vi "TAT_Start.vi"(8 "error In":errorcluster) -> (0 "error out":errorcluster)   [LabVIEW 2017]
uses:
  <vilib>/Utility/error.llb/DialogType.ctl
  Controls/Ass. Loop Control.ctl
  <vilib>/addons/database/Connection.llb/Conn ObjectReference.ctl
  7638e5b4-8d4b-4e71-8911-39d6dd532d8c.vi
  b10198c8-4cf2-4d3c-be81-bfa44f374683.vi
  d2a8d04d-9241-49bb-b773-132ee28ef79b.vi
  f36397dc-6f6c-4e3f-bd29-f8e22a7ab89b.vi
  <vilib>/addons/database/Connection.llb/DB Tools Open Connec (Path).vi
  Global/Global 1.vi
  <vilib>/addons/database/NI_Database_API.lvlib
  <vilib>/Utility/config.llb/NI_LVConfig.lvlib
  user32.dll
panel:
  in  "BARCODE STATION 3":string caption="QR CODE :-"
  out "USER:-":string
  in  "Station Tabs":T1(tab)
  out "PRINT LABEL PICKUP":bool caption="LEAK RESULT:-"
  out "RAREJECTION BIN":bool caption="LEAK RESULT:-"
  out "HBC RH PART SENSOR":bool caption="LEAK RESULT:-"
  out "PY1B RHD RH PART SENSOR":bool caption="LEAK RESULT:-"
  out "PY1B LHD RH PART SENSOR":bool caption="LEAK RESULT:-"
  out "HBC LH PART SENSOR":bool caption="LEAK RESULT:-"
  out "PY1B RHD LH PART SENSOR":bool caption="LEAK RESULT:-"
  out "PY1B LHD LH PART SENSOR":bool caption="LEAK RESULT:-"
  out "AMBIET TEMP MIN":u32
  out "BLINKER CURRENT MAX":u32
  out "TEMP SENSOR MAX":u32
  out "BLINKER CURRENT MIN":u32
  out "TEMP SENSOR MIN":u32
  out "String":string="PARAMETERS"
  out "PART NAME :-":string
  out "QR STATION 3":string caption="QR CODE:-"
  out "PLC STATUS:-":bool
  out "PART No.:-":string
  out "TORISHI CODE:-":string
  out "PROJECT :-":string
  out "CYCLE START:-":bool caption="LEAK RESULT:-"
  out "CYCLE TIME:-":u32
  out "SERIAL NO.:- 2":i32
  out "CYCLE RESULT:-":bool caption="LEAK RESULT:-"
  out "QR STATION 1":string caption="SCAN QR CODE:-"
  out "HARNESS CODE":string
  out "CYCLE STATUS STATION 1":string caption="CYCLE STATUS 1:-"
  out "BLINKER CURRENT OK st 1":u32
  out "TEMP SENSOR st 1":u32
  out "Blinker ct st1":bool caption="LEAK RESULT:-"
  out "Temp Sensor st1":bool caption="LEAK RESULT:-"
  out "AMBIENT TEMP st 1":u32
  out "AVM St1":bool caption="LEAK RESULT:-"
  out "iv3 camera st1":bool caption="LEAK RESULT:-"
  out "SHIFT":u16 caption="SHIFT:-"
  out "GLASS ACTR CT 1 mA st2 MAX":dbl
  out "GLASS ACTR CT 2 mA st2 MAX":dbl
  out "SKY st2  MAX":dbl
  out "INTERNAL (DEG) st2 MAX":dbl
  out "EXTERNAL (DEG) st2 MAX":dbl
  out "GROUND st2 MAX":dbl
  out "POWER FOLD CURENT st2 MAX":dbl
  out "GLASS ACTR CT 1 mA st2 MIN":dbl
  out "GLASS PULL TEST st2 MIN":dbl
  out "GLASS ACTR CT 2 mA st2 MIN":dbl
  out "SKY st2 3 MIN":dbl
  out "INTERNAL (DEG) sT2 MIN":dbl
  out "EXTERNAL (DEG) st2 MIN":dbl
  out "GROUND st2 MIN":dbl
  out "POWER FOLD CURENT st2 MIN":dbl
  out "String 2":string="PARAMETERS"
  out "GLASS ACTR CT 1 mA st2 2":dbl
  out "GLASS PULL TEST st2 2":dbl
  out "GLASS ACTR CT 1 mA st2":bool caption="LEAK RESULT:-"
  out "GLASS PULL TEST st2":bool caption="LEAK RESULT:-"
  out "GLASS ACTR CT 2 mA st 2":dbl
  out "GLASS ACTR CT 2 mA st2":bool caption="LEAK RESULT:-"
  out "SKY st2 2":dbl
  out "INTERNAL (DEG) st2":dbl
  out "SKY st2":bool caption="LEAK RESULT:-"
  out "INTERNAL (DG) st2":bool caption="LEAK RESULT:-"
  out "EXTERNAL (DEG) st2 2":dbl
  out "EXTERNAL (DEG) st2":bool caption="LEAK RESULT:-"
  out "GROUND st 2":dbl
  out "GROUND st2":bool caption="LEAK RESULT:-"
  out "POWER FOLD CURENT st 3":dbl
  out "POWER FOLD CURENT st 2":bool caption="LEAK RESULT:-"
  out "QR STATION 2":string caption="QR CODE:-"
  out "SCAN QR STATION 2":string caption="SCAN QR CODE:-"
  out "CYCLE STATUS STATION 2":string caption="CYCLE STATUS 1:-"
  out "PART No.:- St2":string caption="PART No-"
  out "TORISHI :- St2":string caption="TORISHI-"
  out "PLC STATUS:- 2":bool
  out "PART NAME :- St2":string caption="PART NAME-"
  out "CYCLE RESULT:- St2":bool caption="CYCLE RESULT:-"
  out "SERIAL NO.:- St2":i32 caption="SERIAL NO.:-"
  out "CYCLE TIME:-St2":u32 caption="CYCLE TIME:- 2"
  out "CYCLE START:- St 2":bool caption="LEAK RESULT:-"
  out "PY1B LHD LH PART SENSOR 2":bool caption="LEAK RESULT:-"
  out "PY1B & HBC RH PART VERI SENSR":bool caption="LEAK RESULT:-"
  out "GASKET PRESENT SENSOR 2":bool caption="LEAK RESULT:-"
  out "PY1B LHD RH PART SENSOR 2":bool caption="LEAK RESULT:-"
  out "PY1B & HBC LH PART VERI SENSR":bool caption="LEAK RESULT:-"
  out "GASKET PRESENT SENSOR 1":bool caption="LEAK RESULT:-"
  out "RAREJECTION BIN 2":bool caption="LEAK RESULT:-"
  out "PRINT LABEL PICKUP 2":bool caption="LEAK RESULT:-"
  out "Station 1 Bypass":bool
  out "PACKAGE Qty":string
  out "Scanned Qty  2":string
  out "PREVIOUS BARCODE 2":string[](array[string])
  in  "Model Selection:-":string(combo)
  out "CYCLE STATUS STATION 3":string caption="CYCLE STATUS 2:-"
  out "SCANNED QUANTITY":string
  out "PACKAGED QUANTITY":string
  out "PREVIOUS BARCODE":string
  out "BARCODE STATION 3 only display":string caption="QR CODE :-"
  out "PRN to Print":string
  out "PACKAGE STICKER":string
  in  "Stop":bool
  out "RESULT STATION 1":bool caption="FINAL RESULT:-"
  in  "ASS-Alarms":bool
  out "DATE/TIME":string
  # "Nm"
  # "UNIQUE CIRCLE\nAUTOMATION Pvt Ltd"
  # "MIN"
  # "ACTUAL"
  # "MAX"
  # "RESULT"
  # "AMBIENT TEMP"
  # "AVM"
  # "ARABIC_SIGNAL"
  # "BLINKER CURRENT"
  # "TEMP SENSOR"
  # "ACTUAL"
  # "MIN"
  # "MAX"
  # "RESULT"
  # "GLASS ACTR CT 1 mA"
  # "GLASS PULL TEST"
  # "GLASS ACTR CT 2 mA"
  # "GROUND"
  # "SKY"
  # "INTERNAL (DEG)"
  # "EXTERNAL (DEG)"
  # "POWER FOLD CURENT"
  # "MODEL SELECTION:-"
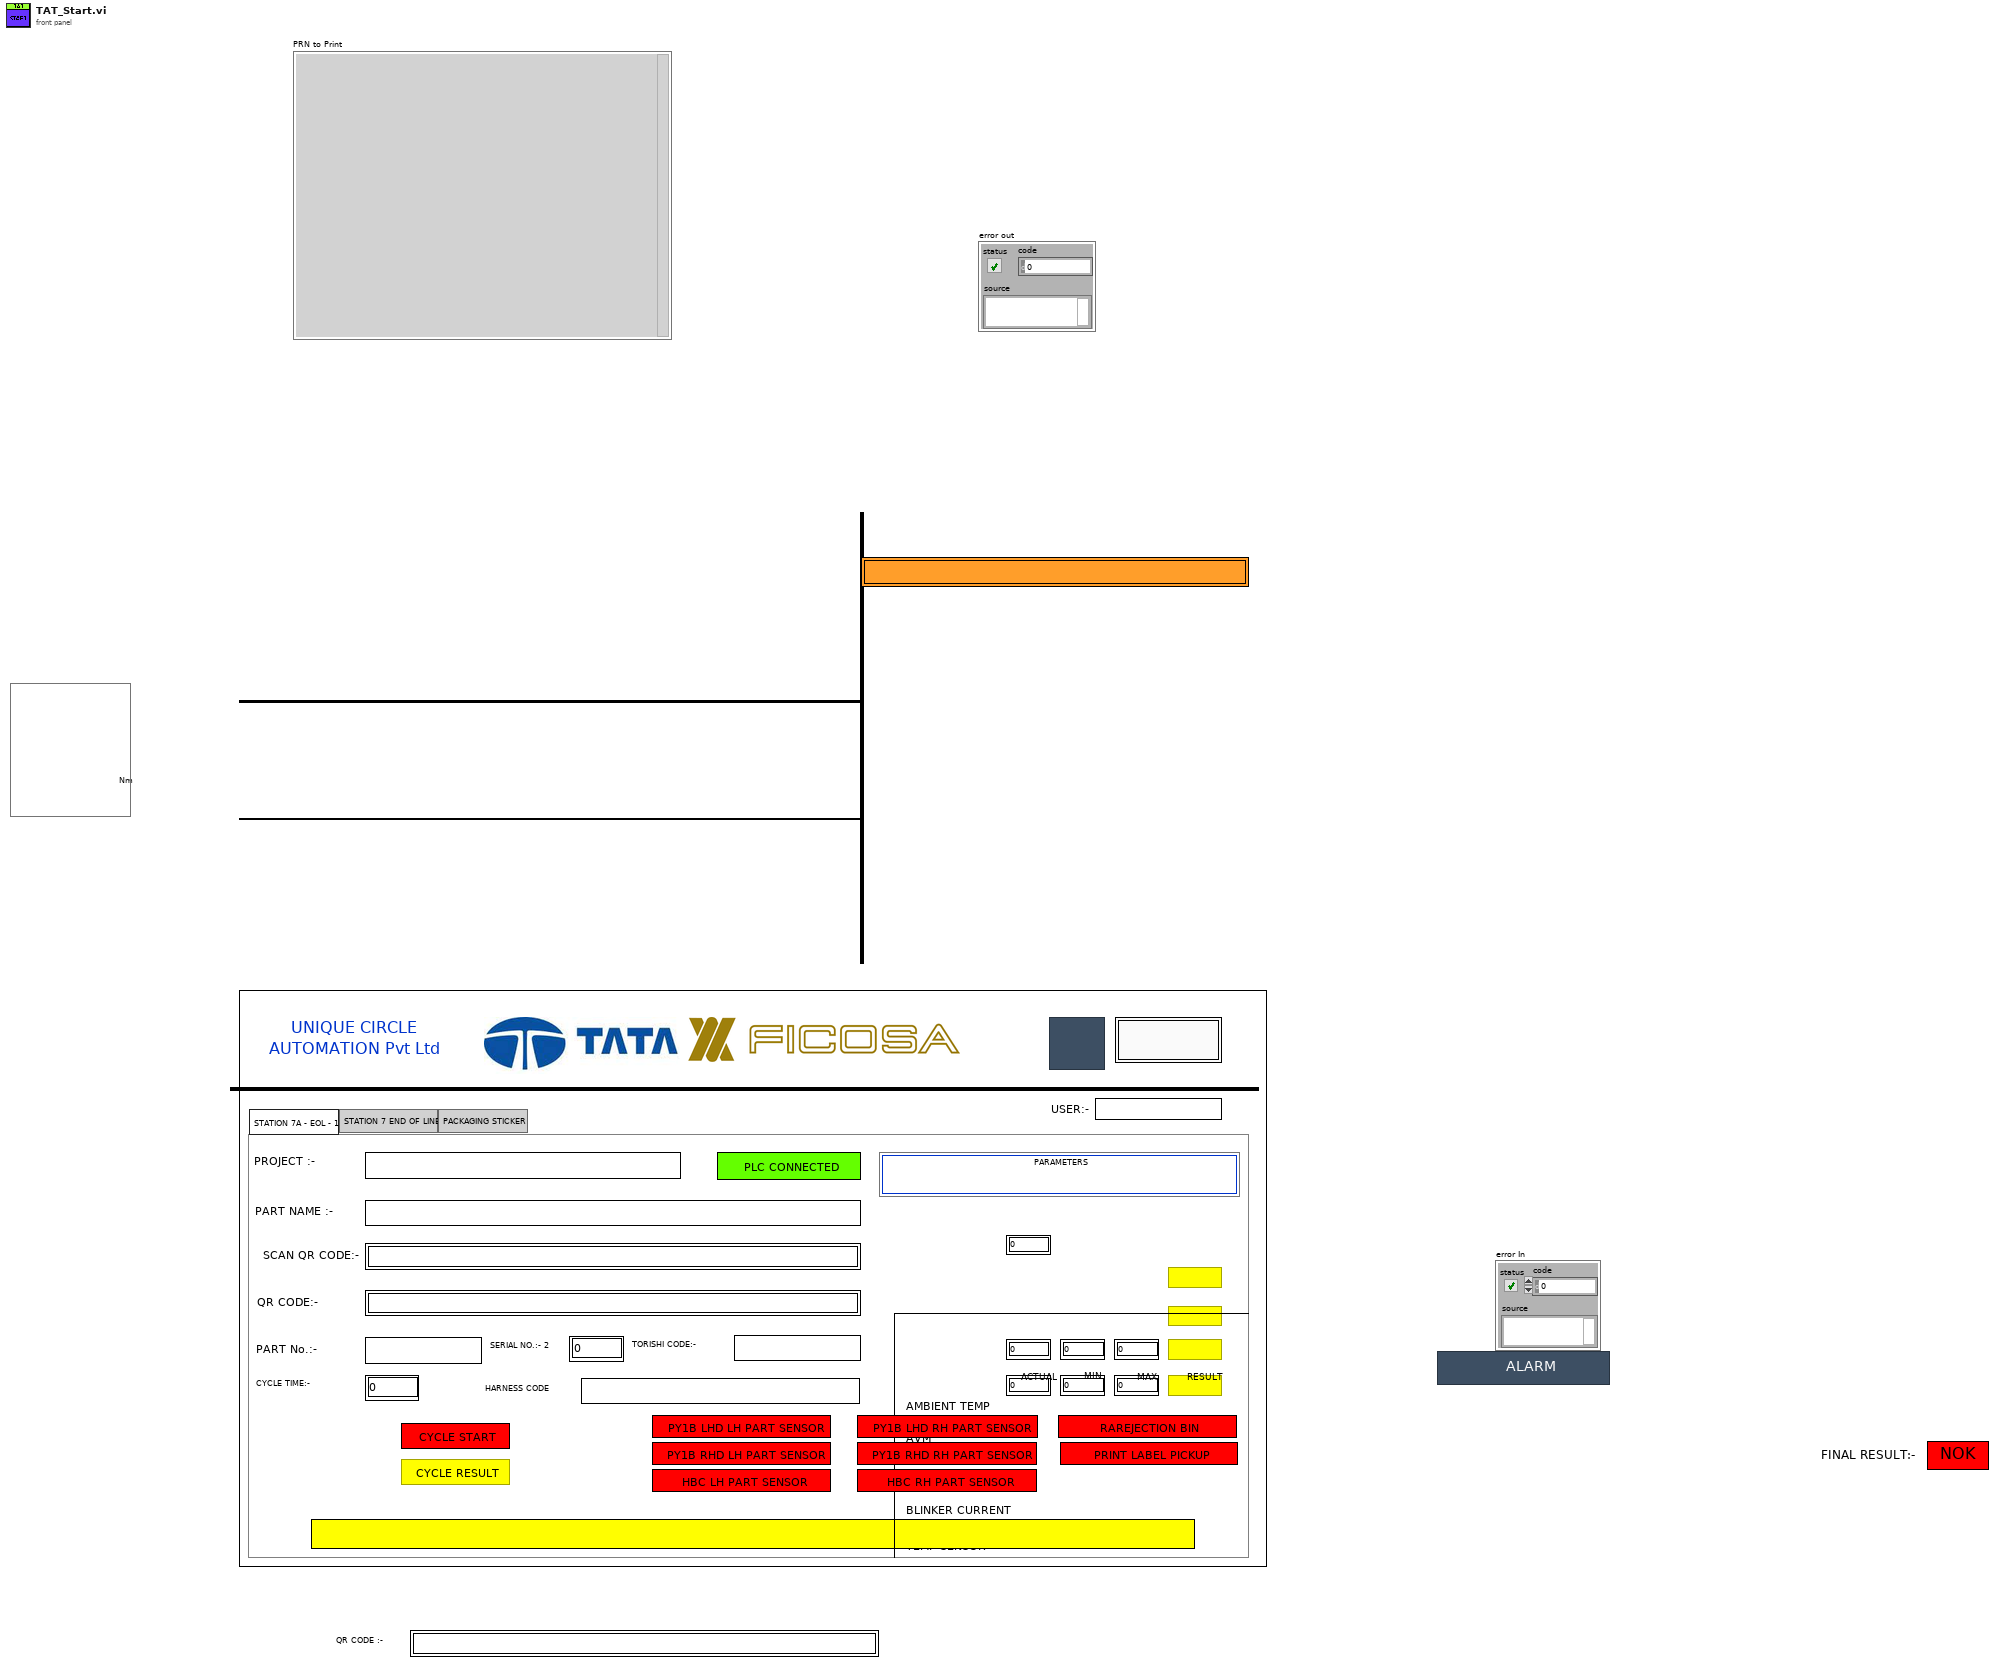
[diagram p1: front panel]
types:
  T1 = enum32{"STATION 7A - EOL - 1", "STATION 7 END OF LINE", "PACKAGING STICKER"}
  T2 = typedef "NI_Database_API.lvlib/Conn ObjectReference.ctl" = refnum<k1>
  T3 = cluster{"Varient number":u16, "Part name":string, "connection reference":T2, "Batch_Size":u16, "PART_NO":string, "TORISHI_CODE":string, "scanner com":refnum<visa-resource-name>, "Part Name List":string[], "Varient path":path, "Current Varient path":path, "Communication path":path, "Package path":path, "Part PRN path":path, "Station2 printer IP":string, "Station1 printer IP":string, "Current Serial Number":string, "Station1_QR":string, "Serial_Number":path, "PREVIOUS code":string[], "Station 2 barcode Dn":string, "Station 2 barcode Up":string, "HARNESS CODE NOT USED":string, "Station 1 bypass":bool}
  T4 = typedef "Ass. Loop Control.ctl" = enum16{"Package_Qty_Count", "GENERATE_QR_PRNT", "Cluster_update", "Waiting_for_scan", "barcode CHECK", "Int", "SaveReport ", "Barcode Print", "Start Cycle", "Wait", "Cycle End", "frontpanel Display update", "Stop"}
  T5 = cluster{"Varient number":u16, "Part name":string, "connection reference":T2, "Batch_Size":u16, "PART_NO":string, "TORISHI_CODE":string, "scanner com":refnum<visa-resource-name>, "Part Name List":string[], "Varient path":path, "Current Varient path":path, "Communication path":path, "Package path":path, "Part PRN path":path, "Station2 printer IP":string, "Station1 printer IP":string, "Current Serial Number":string, "Station2_QR":string, "Serial_Number":path, "PRIVIOUS code":string[], "Barcode station 2 to log Dn":string, "Barcode station 2 to log Up":string, "HARNESS CODE NOT USED":string, "Station1_QR":string, "SearchBitInterlck":bool}
  T6 = cluster{"Varient number":u16, "Part name":string, "Barcode":string, "connection reference":T2, "Batch_Size":u16, "PART_NO":string, "TORISHI_CODE":string, "Varient path":path, "Current Varient path":path, "Communication path":path, "Package path":path, "Part PRN path":path, "Current Serial Number":string, "Station1_QR":string, "Harness_QR_code":string, "SearchBitInterlck":bool}
  T7 = typedef "DialogType.ctl" = u16
  T8 = enum32{"invalid app kind", "Development System", "Run Time System", "Student Edition", "Embedded LabVIEW", "Evaluation", "Custom"}
  T9 = typedef "Semaphore RefNum" = refnum<k1>
  T10 = enum16{"open", "replace", "create", "open or create", "replace or create", "replace or create with confirmation"}
  T11 = cluster{"Varient number":u16, "Part name":string, "connection reference":T2, "Batch_Size":u16, "PART_NO":string, "TORISHI_CODE":string, "scanner com":refnum<visa-resource-name>, "Part Name List":string[], "Varient path":path, "Current Varient path":path, "Communication path":path, "Package path":path, "Part PRN path":path, "Station2 printer IP":string, "Station1 printer IP":string, "Current Serial Number":string, "Station2_QR":string, "Serial_Number":path, "PRIVIOUS code":string[], "Barcode station 2 to log Dn":string, "Barcode station 2 to log Up":string, "HARNESS CODE NOT USED":string, "Station1_QR":string, "searchbitinterlck":bool}
  T12 = typedef "NI_LVConfig.lvlib/Config Data RefNum.ctl" = refnum<k1>
  T13 = cluster{"Varient number":u16, "Part name":string, "Barcode":string, "connection reference":T2, "Batch_Size":u16, "PART_NO":string, "TORISHI_CODE":string, "Varient path":path, "Current Varient path":path, "Communication path":path, "Package path":path, "Part PRN path":path, "Current Serial Number":string, "Station1_QR":string, "Harness_QR_code":string, "searchbitinterlck":bool}
  T14 = cluster{"QR STATION 1":string, "AMBIENT TEMP st 1":u32, "BLINKER CURRENT OK st 1":u32, "TEMP SENSOR st 1":u32}
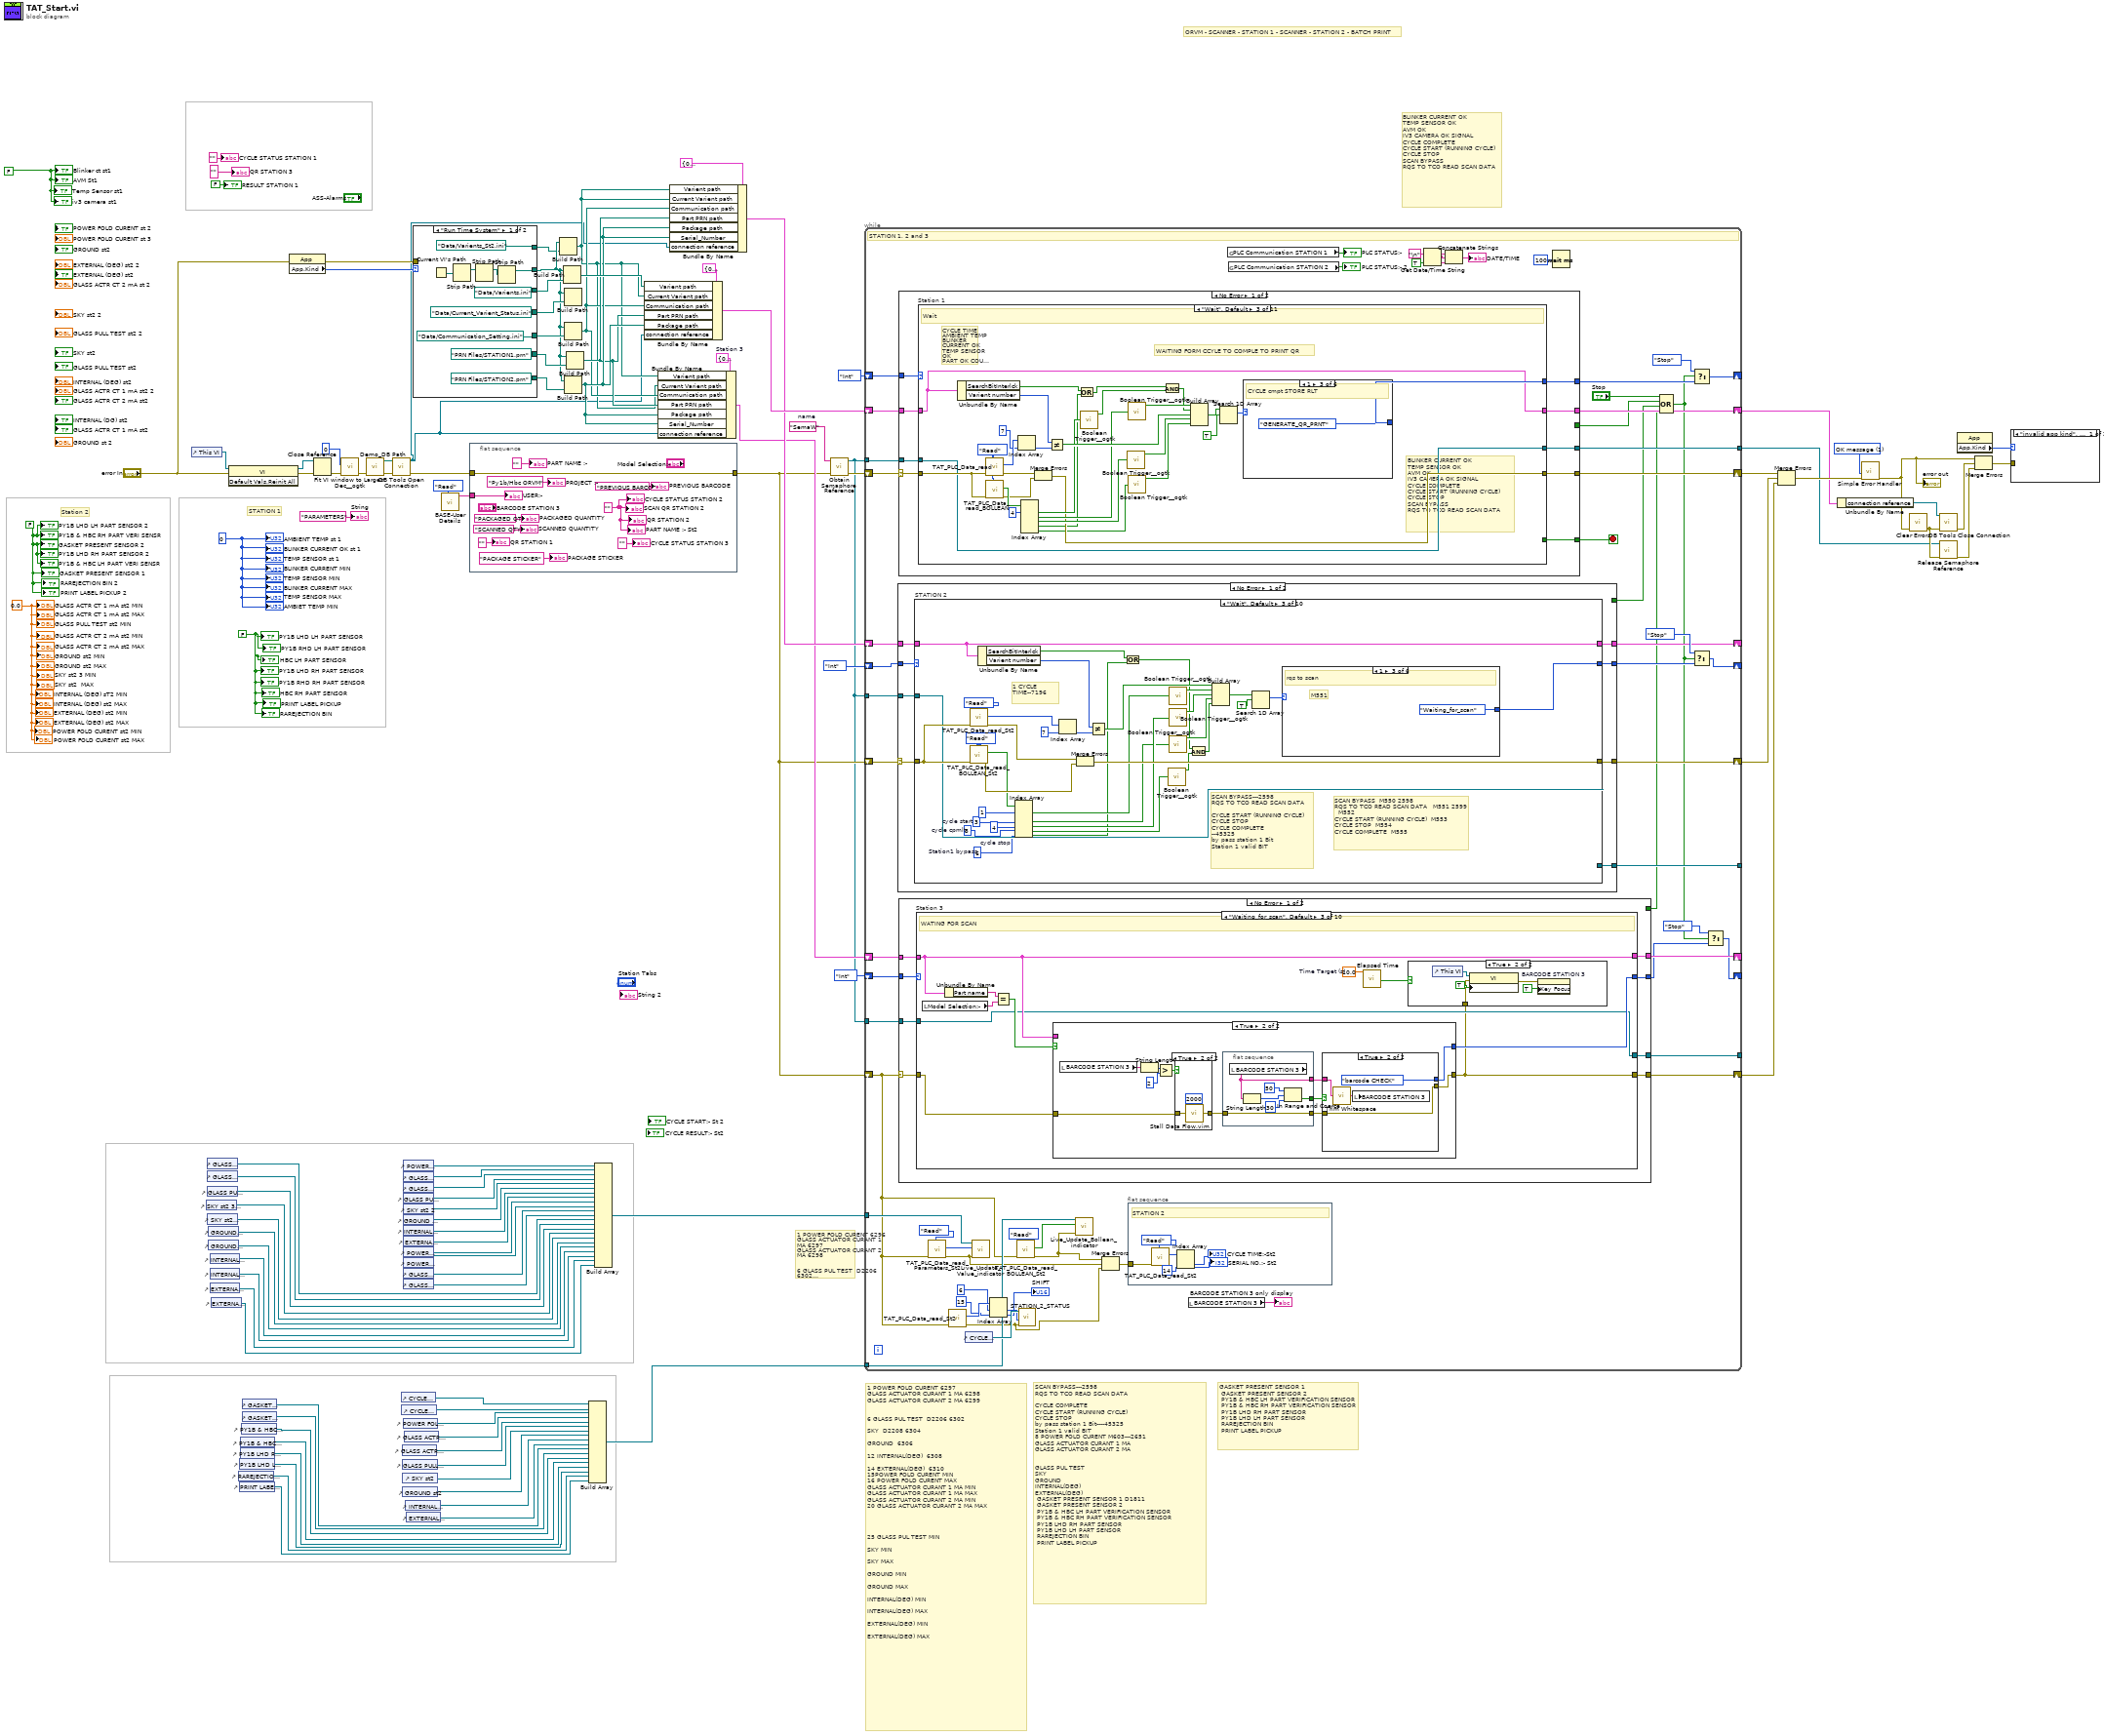
[diagram p0: block diagram]
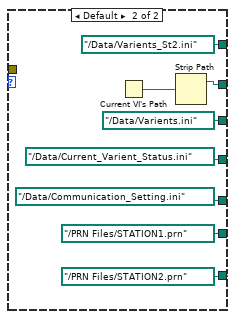
[diagram p2: hidden frame]
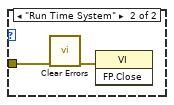
[diagram p3: hidden frame]
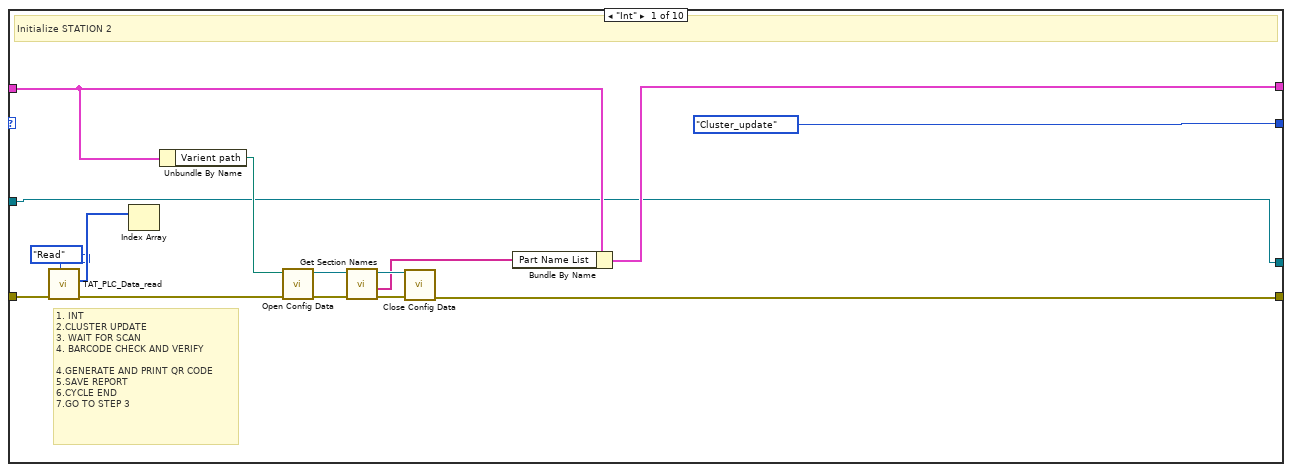
[diagram p4: hidden frame]
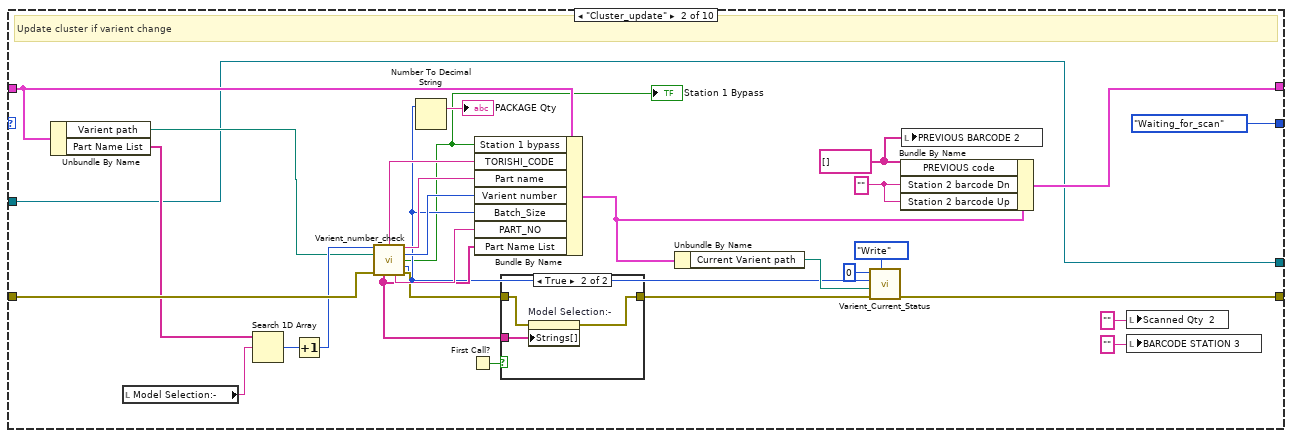
[diagram p5: hidden frame]
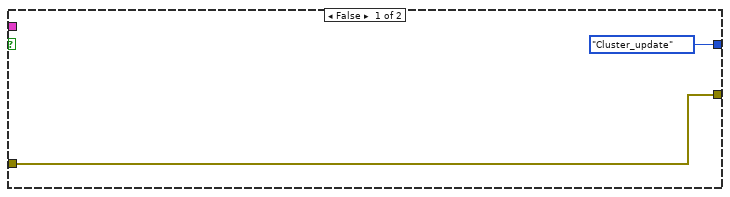
[diagram p8: hidden frame]
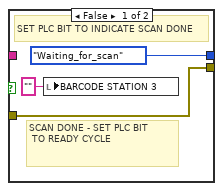
[diagram p10: hidden frame]
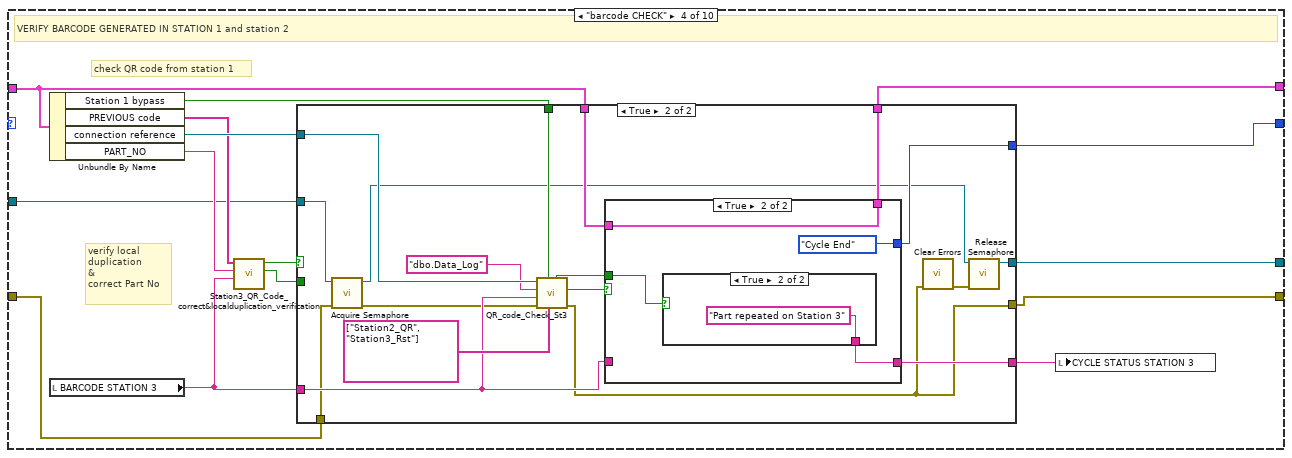
[diagram p11: hidden frame]
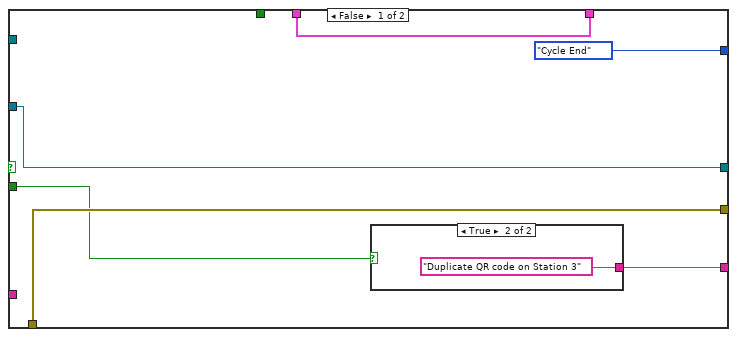
[diagram p12: hidden frame]
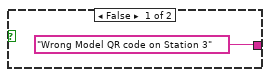
[diagram p13: hidden frame]
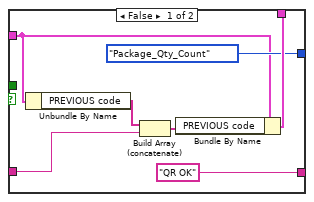
[diagram p14: hidden frame]
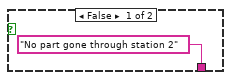
[diagram p15: hidden frame]
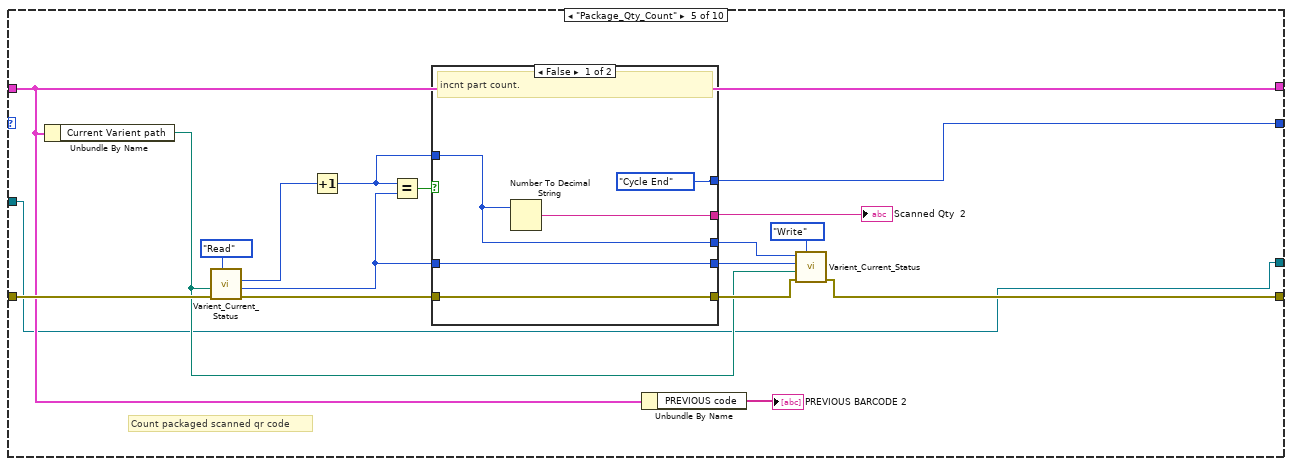
[diagram p16: hidden frame]
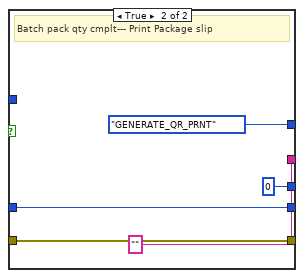
[diagram p17: hidden frame]
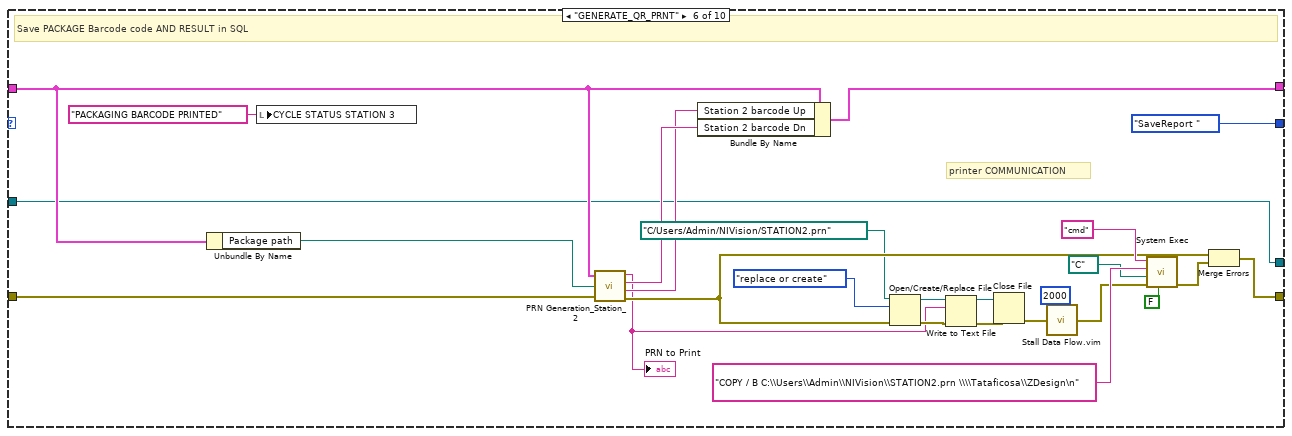
[diagram p18: hidden frame]
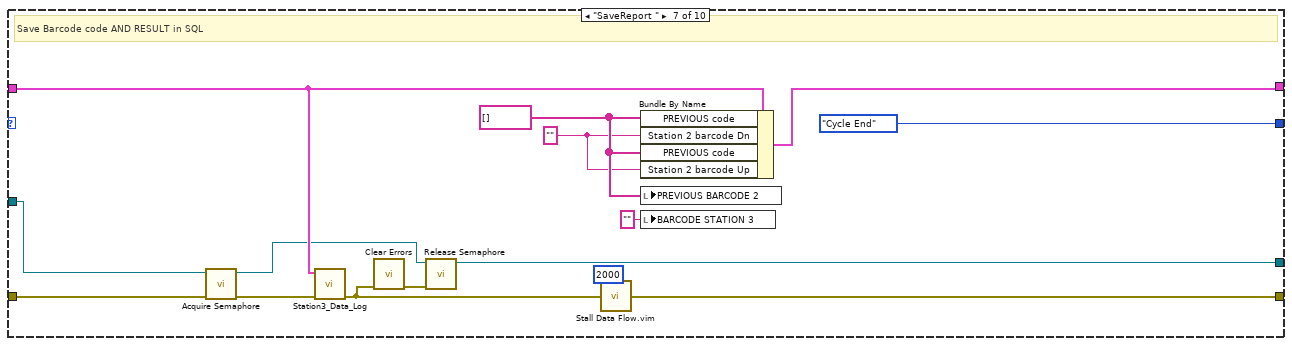
[diagram p19: hidden frame]
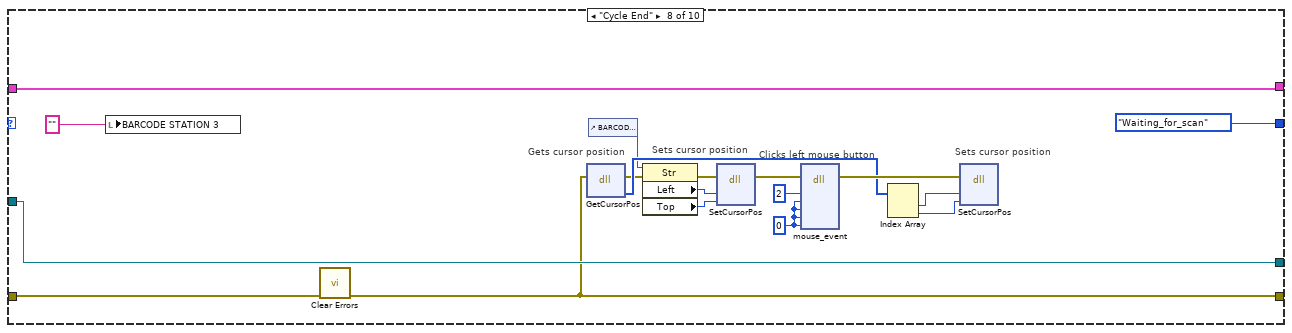
[diagram p20: hidden frame]
diagram:
  w10 = "SemaW"  # name
  w56 = 0.0
  w57 = FALSE
  w58 = FALSE
  w66 = T3 {"Varient number"=0, "Part name"="", "connection reference"=refnum, "Batch_Size"=0, "PART_NO"="", "TORISHI_CODE"="", "scanner com"="", "Part Name List"=[], "Varient path"=path "", "Current Varient path"=path "", "Communication path"=path "", "Package path"=path "", "Part PRN path"=path "", "Station2 printer IP"="", "Station1 printer IP"="", "Current Serial Number"="", "Station1_QR"="", "Serial_Number"=path "", "PREVIOUS code"=[], "Station 2 barcode Dn"="", "Station 2 barcode Up"="", "HARNESS CODE NOT USED"="", "Station 1 bypass"=FALSE}  # Station 3
  w72 = FALSE
  w59 = u32 0 ("AMBIENT TEMP st 1")
  w95 = T7 1 items=["no dialog", "OK message", "continue or stop message", "OK message + warnings", "continue/stop + warnings"] ("type of dialog (OK msg:1)")
  # "GASKET PRESENT SENSOR 1\n GASKET PRESENT SENSOR 2\n PY1B & HBC LH PART VERIFICATION SENSOR\n PY1B & HBC RH PART VERIFICATION SENSOR\n PY1B LHD RH PART SENSOR\n PY1B LHD LH PART SENSOR\n RAREJECTION BIN\n PRINT LABEL PICKUP"
  # "SCAN BYPASS---2598\nRQS TO TCO READ SCAN DATA \n\nCYCLE COMPLETE\nCYCLE START (RUNNING CYCLE)\nCYCLE STOP\nby pass station 1 Bit----45325\nStation 1 valid BIT\n8 POWER FOLD CURENT M603---2651\nGLASS ACTUATOR CURANT 1 MA\nGLASS ACTUATOR CURANT 2 MA\n\n\nGLASS PUL TEST\nSKY \nGROUND\nINTERNAL(DEG)\nEXTERNAL(DEG)\n GASKET PRESENT SENSOR 1 D1811\n GASKET PRESENT SENSOR 2\n PY1B & HBC LH PART VERIFICATION SENSOR\n PY1B & HBC RH PART VERIFICATION SENSOR\n PY1B LHD RH PART SENSOR\n PY1B LHD LH PART SENSOR\n RAREJECTION BIN\n PRINT LABEL PICKUP"
  # "1 POWER FOLD CURENT 6297\nGLASS ACTUATOR CURANT 1 MA 6298\nGLASS ACTUATOR CURANT 2 MA 6299\n\n\n6 GLASS PUL TEST  D2206 6302\n\nSKY  D2208 6304\n\nGROUND  6306\n\n12 INTERNAL(DEG)  6308\n\n14 EXTERNAL(DEG)  6310\n15POWER FOLD CURENT MIN\n16 POWER FOLD CURENT MAX\nGLASS ACTUATOR CURANT 1 MA MIN\nGLASS ACTUATOR CURANT 1 MA MAX\nGLASS ACTUATOR CURANT 2 MA MIN\n20 GLASS ACTUATOR CURANT 2 MA MAX\n\n\n\n\n25 GLASS PUL TEST MIN\n\nSKY MIN\n\nSKY MAX\n\nGROUND MIN\n\nGROUND MAX\n\nINTERNAL(DEG) MIN\n\nINTERNAL(DEG) MAX\n\nEXTERNAL(DEG) MIN\n\nEXTERNAL(DEG) MAX"
  # "Station 2"
  # "STATION 1"
  # "1 POWER FOLD CURENT 6296\nGLASS ACTUATOR CURANT 1 MA 6297\nGLASS ACTUATOR CURANT 2 MA 6298\n\n\n6 GLASS PUL TEST  D2206 6302\n\nSKY  D2208 6304\n\nGROUND  6306\n\n12 INTERNAL(DEG)  6308\n\n14 EXTERNAL(DEG)  6310"
  # "BLINKER CURRENT OK\nTEMP SENSOR OK\nAVM OK\nIV3 CAMERA OK SIGNAL\nCYCLE COMPLETE\nCYCLE START (RUNNING CYCLE)\nCYCLE STOP\nSCAN BYPASS\nRQS TO TCO READ SCAN DATA"
  # "ORVM - SCANNER - STATION 1 - SCANNER - STATION 2 - BATCH PRINT"
  n1 = control-ref of="This VI"() -> (w106:refnum<vi>)
  n2 = control-ref of="SKY st2 3 MIN"() -> (w40:refnum<vi>)
  n3 = control-ref of="GLASS ACTR CT 2 mA st2 MIN"() -> (w43:refnum<vi>)
  n4 = control-ref of="GLASS ACTR CT 2 mA st2 MAX"() -> (w42:refnum<vi>)
  n5 = control-ref of="GLASS PULL TEST st2 MIN"() -> (w41:refnum<vi>)
  n6 = control-ref of="SKY st2  MAX"() -> (w39:refnum<vi>)
  n7 = control-ref of="GROUND st2 MIN"() -> (w38:refnum<vi>)
  n8 = control-ref of="GROUND st2 MAX"() -> (w37:refnum<vi>)
  n9 = control-ref of="INTERNAL (DEG) sT2 MIN"() -> (w36:refnum<vi>)
  n10 = control-ref of="INTERNAL (DEG) st2 MAX"() -> (w35:refnum<vi>)
  n11 = control-ref of="EXTERNAL (DEG) st2 MIN"() -> (w34:refnum<vi>)
  n12 = control-ref of="EXTERNAL (DEG) st2 MAX"() -> (w33:refnum<vi>)
  n13 = invoke class="VI" method="Default Vals.Reinit All"(reference=w106, error in="error In") -> (reference out=w104:refnum<vi>, error out=w105:errorcluster)  [unwired: 1 in, 1 out]
  n14 = control-ref of="RAREJECTION BIN 2"() -> (w15:refnum<vi>)
  n15 = control-ref of="PY1B LHD LH PART SENSOR 2"() -> (w16:refnum<vi>)
  n16 = control-ref of="PRINT LABEL PICKUP 2"() -> (w14:refnum<vi>)
  n17 = control-ref of="PY1B & HBC RH PART VERI SENSR"() -> (w18:refnum<vi>)
  n18 = control-ref of="PY1B LHD RH PART SENSOR 2"() -> (w17:refnum<vi>)
  n19 = control-ref of="PY1B & HBC LH PART VERI SENSR"() -> (w19:refnum<vi>)
  n20 = control-ref of="GASKET PRESENT SENSOR 1"() -> (w21:refnum<vi>)
  n21 = control-ref of="GASKET PRESENT SENSOR 2"() -> (w20:refnum<vi>)
  n22 = property class="App"(error in="error In") -> (error out=w87:errorcluster, "App.Kind"=w92:T8)  [unwired: 1 in, 1 out]
  n23 = Close Reference(reference=w104, error in (no error)=w105) -> (error out=w103:errorcluster)
  n24 = call <userlib>:"Fit VI window to Largest Dec__ogtk.vi"("error in (no error)"=w103, "border spacing (2 px)"=0) -> ("error out"=w80:errorcluster)  [unwired: 4 in, 1 out]
  n25 = call "Demo_DB Path.vi"("error in"=w80) -> ("error out"=w82:errorcluster, "DB Path"=w81:path)  [unwired: 9 in]
  n26 = call-poly <vilib>:"DB Tools Open Connection.vi"("error in (no error)"=w82, "connection information"=w81) -> ("error out"=w4:errorcluster, "connection reference"=w3:T2)  [unwired: 6 in]
  n27 = control-ref of="CYCLE START:- St 2"() -> (w31:refnum<vi>)
  n28 = control-ref of="CYCLE RESULT:- St2"() -> (w30:refnum<vi>)
  n29 = control-ref of="GLASS ACTR CT 2 mA st2"() -> (w27:refnum<vi>)
  n30 = control-ref of="GLASS PULL TEST st2"() -> (w26:refnum<vi>)
  n31 = control-ref of="SKY st2"() -> (w25:refnum<vi>)
  n32 = control-ref of="GROUND st2"() -> (w24:refnum<vi>)
  n33 = control-ref of="POWER FOLD CURENT st 3"() -> (w55:refnum<vi>)
  n34 = control-ref of="GLASS ACTR CT 1 mA st2 2"() -> (w54:refnum<vi>)
  n35 = control-ref of="GLASS ACTR CT 2 mA st 2"() -> (w53:refnum<vi>)
  n36 = control-ref of="GLASS PULL TEST st2 2"() -> (w52:refnum<vi>)
  n37 = control-ref of="SKY st2 2"() -> (w51:refnum<vi>)
  n38 = control-ref of="GROUND st 2"() -> (w50:refnum<vi>)
  n39 = control-ref of="INTERNAL (DEG) st2"() -> (w49:refnum<vi>)
  n40 = control-ref of="EXTERNAL (DEG) st2 2"() -> (w48:refnum<vi>)
  n41 = control-ref of="POWER FOLD CURENT st2 MIN"() -> (w47:refnum<vi>)
  n42 = control-ref of="POWER FOLD CURENT st2 MAX"() -> (w46:refnum<vi>)
  n43 = control-ref of="GLASS ACTR CT 1 mA st2 MIN"() -> (w45:refnum<vi>)
  n44 = control-ref of="GLASS ACTR CT 1 mA st2 MAX"() -> (w44:refnum<vi>)
  n45 = control-ref of="POWER FOLD CURENT st 2"() -> (w29:refnum<vi>)
  n46 = control-ref of="GLASS ACTR CT 1 mA st2"() -> (w28:refnum<vi>)
  n47 = control-ref of="INTERNAL (DG) st2"() -> (w23:refnum<vi>)
  n48 = control-ref of="EXTERNAL (DEG) st2"() -> (w22:refnum<vi>)
  n49 = case shown="\"Run Time System\"" w92 {
    tunnel: [path "Data/Varients.ini" ("path") path "../Data/Varients.ini" ("path")] -> w91
    tunnel: [w112 w122] -> w69
    tunnel: [path "Data/Current_Varient_Status.ini" ("path") path "../Data/Current_Varient_Status.ini" ("path")] -> w90
    tunnel: [path "Data/Communication_Setting.ini" ("path") path "../Data/Communication_Setting.ini" ("path")] -> w89
    tunnel: [path "PRN Files/STATION2.prn" ("path") path "../PRN Files/STATION2.prn" ("path")] -> w88
    tunnel: w87 -> [_ _]
    tunnel: [path "PRN Files/STATION1.prn" ("path") path "../PRN Files/STATION1.prn" ("path")] -> w85
    tunnel: [path "Data/Varients_St2.ini" ("path") path "../Data/Varients_St2.ini" ("path")] -> w68
    frame "Run Time System" {
      n50 = Current VI's Path() -> (path=w115:path)
      n51 = Strip Path(path=w115) -> (stripped path=w114:path)  [unwired: 1 out]
      n52 = Strip Path(path=w114) -> (stripped path=w113:path)  [unwired: 1 out]
      n53 = Strip Path(path=w113) -> (stripped path=w112:path)  [unwired: 1 out]
    }
    frame Default {
      n54 = Current VI's Path() -> (path=w123:path)
      n55 = Strip Path(path=w123) -> (stripped path=w122:path)  [unwired: 1 out]
    }
  }
  n56 = call "BASE-User Details.vi"("Enum"=enum16{"Read", "Write"}."Read") -> ("User Name Out"=w96:string)  [unwired: 9 in, 1 out]
  n57 = flat-sequence {
    tunnel: [w135] -> w12
    tunnel: w4 -> [w135]
    tunnel: w96 -> [w133]
    frame #0 {
      w125 = "" ("BARCODE STATION 2")
      "USER:-" <- w133
      "PART NAME :-" <- ""
      "PROJECT :-" <- "Py1b/Hbc ORVM" ("PROJECT")
      "CYCLE STATUS STATION 3" <- "" ("CYCLE STATUS STATION 2")
      "PACKAGE STICKER" <- "PACKAGE STICKER" ("PACKAGE STICKER")
      "SCANNED QUANTITY" <- "SCANNED QTY" ("PACKAGE STICKER")
      "PACKAGED QUANTITY" <- "PACKAGED QTY" ("PACKAGE STICKER")
      "PREVIOUS BARCODE" <- "PREVIOUS BARCODE" ("PACKAGE STICKER")
      "QR STATION 1" <- "" ("BARCODE STATION 2")
      "SCAN QR STATION 2" <- w125
      "QR STATION 2" <- w125
      "CYCLE STATUS STATION 2" <- w125
      "PART NAME :- St2" <- w125
    }
  }
  n58 = Build Path(base path=w69, name or relative path=w68) -> (appended path=w61:path)
  n59 = Build Path(base path=w69, name or relative path=w91) -> (appended path=w67:path)
  n60 = Build Path(base path=w69, name or relative path=w90) -> ()  [unwired: 1 out]
  n61 = Build Path(base path=w69, name or relative path=w88) -> (appended path=w65:path)
  n62 = Build Path(base path=w69, name or relative path=w89) -> (appended path=w63:path)
  n63 = Build Path(base path=w69, name or relative path=w85) -> (appended path=w64:path)
  n64 = Build Array(w31, w30, w29, w28, w27, w26, w25, w24, w23, w22, w21, w20, w19, w18, w17, w16, w15, w14) -> (w13:refnum<vi>[])
  n65 = Build Array(w55, w54, w53, w52, w51, w50, w49, w48, w47, w46, w45, w44, w43, w42, w41, w40, w39, w38, w37, w36, w35, w34, w33) -> (w32:refnum<vi>[])
  n66 = Bundle By Name(cluster=T6 {"Varient number"=0, "Part name"="", "Barcode"="", "connection reference"=refnum, "Batch_Size"=0, "PART_NO"="", "TORISHI_CODE"="", "Varient path"=path "", "Current Varient path"=path "", "Communication path"=path "", "Package path"=path "", "Part PRN path"=path "", "Current Serial Number"="", "Station1_QR"="", "Harness_QR_code"="", "SearchBitInterlck"=FALSE}, "Varient path"=w67, "Current Varient path"=w61, "Communication path"=w63, "Part PRN path"=w64, "Package path"=w65, "connection reference"=w3) -> (w83:T6)
  n67 = Bundle By Name(cluster=w66, "Varient path"=w61, "Current Varient path"=w61, "Communication path"=w63, "Part PRN path"=w64, "Package path"=w65, "Serial_Number"=w65, "connection reference"=w3) -> (w62:T3)
  n68 = Bundle By Name(cluster=T5 {"Varient number"=0, "Part name"="", "connection reference"=refnum, "Batch_Size"=0, "PART_NO"="", "TORISHI_CODE"="", "scanner com"="", "Part Name List"=[], "Varient path"=path "", "Current Varient path"=path "", "Communication path"=path "", "Package path"=path "", "Part PRN path"=path "", "Station2 printer IP"="", "Station1 printer IP"="", "Current Serial Number"="", "Station2_QR"="", "Serial_Number"=path "", "PRIVIOUS code"=[], "Barcode station 2 to log Dn"="", "Barcode station 2 to log Up"="", "HARNESS CODE NOT USED"="", "Station1_QR"="", "SearchBitInterlck"=FALSE}, "Varient path"=w61, "Current Varient path"=w61, "Communication path"=w63, "Part PRN path"=w64, "Package path"=w65, "Serial_Number"=w65, "connection reference"=w3) -> (w71:T5)
  n69 = call <vilib>:"Obtain Semaphore Reference.vi"("error in (no error)"=w12, "name (unnamed)"=w10) -> ("error out"=w11:errorcluster, "semaphore"=w9:T9)  [unwired: 3 in, 1 out]
  n70 = while {
    shift-right: [w193] -> _
    shift-left: Ass._Loop_Control."Int" ("Enum") -> [w196]
    shift-right: [w180] -> w78
    shift-left: w83 -> [w194]
    shift-right: [w182] -> _
    shift-left: Ass._Loop_Control."Int" ("Enum") -> [w185]
    shift-right: [w183] -> _
    shift-left: w62 -> [w184]
    shift-right: [w175] -> _
    shift-left: Ass._Loop_Control."Int" ("Enum") -> [w178]
    shift-right: [w174] -> _
    shift-left: w71 -> [w173]
    shift-right: [w163] -> w6
    shift-left: w12 -> [w157]
    tunnel: w32 -> [w159]
    tunnel: w13 -> [w158]
    tunnel: w9 -> [w150]
    tunnel: [w149] -> w7
    tunnel: w9 -> [w148]
    tunnel: [w147] -> _
    tunnel: w9 -> [w146]
    tunnel: [w145] -> _
    shift-right: [w151] -> w2
    shift-left: w12 -> [w179]
    shift-right: [w152] -> w1
    shift-left: w11 -> [w139]
    stop <- w186 stop-if-true
    # "STATION 1, 2 and 3"
    n71 = case shown="No Error" w179 {
      selector: w179 -> [w465 w810]
      tunnel: w178 -> [w464 _]
      tunnel: [w463 w813] -> w176
      tunnel: [w462 w814] -> w174
      tunnel: w173 -> [w461 w814]
      tunnel: [w460 w808] -> w151
      tunnel: w148 -> [w459 w812]
      tunnel: [w458 w812] -> w147
      tunnel: [_ TRUE] -> w141
      frame No Error {
        n72 = case "STATION 2" shown="\"Wait\", Default" w464 {
          tunnel: [Ass._Loop_Control."Cluster_update" ("Enum") Ass._Loop_Control."Wait" ("Enum") w529 Ass._Loop_Control."barcode CHECK" ("Enum") w588 Ass._Loop_Control."Wait" ("Enum") Ass._Loop_Control."SaveReport " ("Enum") Ass._Loop_Control."Cycle End" ("Enum") Ass._Loop_Control."Wait" ("Enum") Ass._Loop_Control."Stop" ("Enum")] -> w463
          tunnel: [w487 w502 w530 w573 w575 w706 w717 w745 w754 w802] -> w462
          tunnel: [w483 w506 w542 w557 w585 w689 w716 w738 w761 w785] -> w460
          tunnel: w465 -> [w484 w501 w526 w558 w591 w704 w715 w744 w765 w799]
          tunnel: w461 -> [w487 w505 w530 w573 w584 w706 w725 w745 w755 w802]
          tunnel: w459 -> [w482 w492 w518 w554 w578 w702 w712 w735 w762 w783]
          tunnel: [w482 w492 w518 w554 w577 w702 w712 w733 w762 w783] -> w458
          frame "Int" {
            w466 = enum16{"update", "init"}."init"  # Enum
            w467 = "initia"  # Log data
            # "Keep this on as in first cycle this bit need to be ON.\nRQST FROM TCO RESET SCAN DATA\tM545\t\t\t2593"
            # "SCAN OK\tM542\t\t\t2590\nSCAN NG \tM543\t\t\t2591\nSoftware on Bit\tM544\t\t\t2592\nRQST FROM TCO RESET SCAN DATA\tM545\t\t\t2593\nRepeat scan part\t\tM547\t\t2595\nPass not done station 1\t\tM548\t\t2596"
            # "Initialize STATION 2"
            n73 = control-ref of="CYCLE STATUS STATION 2"() -> (w485:refnum<vi>)
            n74 = call "STATION_2_STATUS.vi"("error in (no error)"=w484, "STATUS"="STATION 7 END OF LINE" ("TexT"), "Ctl Refnum"=w485) -> ("error out"=w469:errorcluster)  [unwired: 8 in]
            n75 = call "TAT_LABVIEW_TO_PLC_St2.vi"("Enum"=enum16{"Read", "Write"}."Read", "error in (no error)"=w469) -> ("error out"=w480:errorcluster, "Array 2"=w473:bool[])  [unwired: 8 in]
            n76 = in-place {
              in-place-border: [w491] -> w481
              in-place-border: w480 -> [w491]
              w490 = FALSE ("element")
              w489 = TRUE ("new element/subarray")
              n77 = in-place-array #1(w473, 0, 1, 2, 3, 4, 5) -> ()  [unwired: 6 out]
              n78 = in-place-array #1(w490, w490, w489, w489, w490, w490) -> (w478:bool[])  [unwired: 6 out]
            }
            n79 = call "TAT_LABVIEW_TO_PLC_St2.vi"("Enum"=enum16{"Read", "Write"}."Write", "error in (no error)"=w481, "Array"=w478) -> ("error out"=w468:errorcluster)  [unwired: 7 in, 1 out]
            n80 = Merge Errors(w468) -> (w483:errorcluster)
            n81 = call "debuglog.vi"("Enum"=w466, "Log data"=w467) -> ()  [unwired: 10 in]
          }
          frame "Cluster_update" {
            # "Update cluster if varient change"
            n82 = call "TAT_PLC_Data_read_St2.vi"("Enum"=enum16{"Read", "Write"}."Read", "error in (no error)"=w501) -> ("error out"=w500:errorcluster, "Array 2"=w497:u16[])  [unwired: 8 in]
            n83 = Unbundle By Name(w505) -> ("Varient path"=w507:path)
            n84 = Index Array(array=w497, index=7) -> (element=w496:u16)
            n85 = call "Varient_number_check.vi"("Varient No."=w496, "Varient path"=w507, "error in"=w500) -> ("TORISHI_CODE"=w494:string, "Part Name"=w493:string, "Varient Number"=w504:i32, "Batch Size"=w503:i32, "PART_NO"=w495:string, "error out"=w506:errorcluster)  [unwired: 4 in, 3 out]
            "PART No.:- St2" <- w495
            "TORISHI :- St2" <- w494
            n86 = local write "PART NAME :- St2"(w493) -> ()
            n87 = Bundle By Name(cluster=w505, "TORISHI_CODE"=w494, "Part name"=w493, "Varient number"=w504, "Batch_Size"=w503, "PART_NO"=w495) -> (w502:T5)
          }
          frame "Wait", Default {
            w511 = 6  # Station1 bypass
            w515 = 5  # cycle cpmlt
            w516 = 4  # cycle stop
            w517 = 3  # cycle start
            # "SCAN BYPASS\t\tM550\t2598\nRQS TO TCO READ SCAN DATA \t\tM551\t2599\n\t\tM552\t\nCYCLE START (RUNNING CYCLE)\t\tM553\t\nCYCLE STOP\t\tM554\t\nCYCLE COMPLETE\t\tM555"
            # "SCAN BYPASS---2598\nRQS TO TCO READ SCAN DATA \n\nCYCLE START (RUNNING CYCLE)\nCYCLE STOP\nCYCLE COMPLETE\n--45325\nby pass station 1 Bit\nStation 1 valid BIT"
            # "1 CYCLE TIME--7196\n\n\n\n\n\n7 FAULT BIT ----4356\nVARIENT\nHOUR\nMINUTE\nSECOND\nDAY\nMONTH\nYEAR\nSERIAL NUMBER\nShift\nPOWER FOLD ACTUATO--D6061\nGLASS ACTUATOR 1 &2"
            n88 = call "TAT_PLC_Data_read_BOLLEAN_St2.vi"("Enum"=enum16{"Read", "Write"}."Read", "error in (no error)"=w526) -> ("error out"=w543:errorcluster, "Array 2"=w522:bool[])  [unwired: 8 in]
            n89 = call "TAT_PLC_Data_read_St2.vi"("Enum"=enum16{"Read", "Write"}."Read", "error in (no error)"=w526) -> ("error out"=w525:errorcluster, "Array 2"=w527:u16[])  [unwired: 8 in]
            n90 = Unbundle By Name(w530) -> ("SearchBitInterlck"=w510:bool, "Varient number"=w536:u16)
            n91 = Index Array(array=w522, index #1=1 ("index"), index #3=w517, index #4=w516, index #5=w515, index #6=w511) -> (element #1=w523:bool, element #3=w519:bool, element #4=w520:bool, element #5=w521:bool, element #6=w512:bool)  [unwired: 1 in, 1 out]
            n92 = Index Array(array=w527, index=7) -> (element=w535:u16)
            n93 = Merge Errors(w525, w543) -> (w542:errorcluster)
            n94 = Not Equal?(x=w536, y=w535) -> (x != y?=w524:bool)
            n95 = Or(x=w510, y=w512) -> (x .or. y?=w509:bool)
            n96 = call <userlib>:"Boolean Trigger__ogtk.vi"("Boolean Input"=w521) -> ("Rising Edge"=w514:bool)  [unwired: 1 in, 1 out]
            n97 = call <userlib>:"Boolean Trigger__ogtk.vi"("Boolean Input"=w519) -> ("Rising Edge"=w540:bool)  [unwired: 1 in, 1 out]
            n98 = call <userlib>:"Boolean Trigger__ogtk.vi"("Boolean Input"=w523) -> ("Rising Edge"=w532:bool)  [unwired: 1 in, 1 out]
            n99 = call <userlib>:"Boolean Trigger__ogtk.vi"("Boolean Input"=w520) -> ("Rising Edge"=w537:bool)  [unwired: 1 in, 1 out]
            n100 = And(x=w509, y=w514) -> (x .and. y?=w513:bool)
            n101 = Build Array(w524, w532, w537, w540, w513) -> (w533:bool[])
            n102 = Search 1D Array(1D array=w533, element=TRUE ("Boolean Input")) -> (index of element=w534:i32)  [unwired: 1 in]
            n103 = case shown="1" w534 {
              tunnel: [Ass._Loop_Control."Wait" ("Enum") Ass._Loop_Control."Cluster_update" ("Enum") Ass._Loop_Control."Waiting_for_scan" ("Enum") Ass._Loop_Control."Cycle End" ("Enum") Ass._Loop_Control."Start Cycle" ("Enum") Ass._Loop_Control."GENERATE_QR_PRNT" ("Enum")] -> w529
              frame -1, Default {
              }
              frame 0 {
                # "cluster update"
              }
              frame 1 {
                # "M551"
                # "rqs to scan"
              }
              frame 2 {
                w547 = enum16{"update", "init"}."update"  # Enum
                w548 = "direct cycle stop"  # Log data
                # "M554"
                # "E-Stops"
                # "cycle Stop"
                n104 = call "debuglog.vi"("Enum"=w547, "Log data"=w548) -> ()  [unwired: 10 in]
              }
              frame 3 {
                # "M553"
                # "cycle start"
              }
              frame 4 {
                # "M555"
                # "cycle cmplt"
              }
            }
          }
          frame "Waiting_for_scan" {
            w552 = enum16{"update", "init"}."update"  # Enum
            w553 = "search bit rcv"  # Log data
            # "WATING FOR SCAN"
            n105 = call "Station 2 QR Code.vi"("Enum"=enum16{"Read", "Write"}."Read", "error in (no error)"=w558) -> ("error out"=w557:errorcluster, "Array 2"=w561:u16[])  [unwired: 8 in]
            n106 = Type Cast(type="", x=w561) -> (*(type *) &x=w571:string)
            n107 = String Subset(string=w571, length (rest)=49 ("length (rest)")) -> (substring=w572:string)  [unwired: 1 in]
            n108 = call <vilib>:"Space Constant.vi"() -> ("String"=w568:string)
            n109 = Search and Replace String(replace all?=TRUE ("replace all? (F)"), input string=w572, search string="[^a-zA-Z0-9/]", replace string=w568) -> (result string=w569:string)  [unwired: 4 in, 3 out]
            n110 = call <vilib>:"Trim Whitespace.vi"("string"=w569) -> ("trimmed string"=w570:string)  [unwired: 1 in]
            n111 = Search and Replace String(replace all?=TRUE ("replace all? (F)"), input string=w570, search string="  ", replace string=" " ("search string")) -> (result string=w556:string)  [unwired: 4 in, 3 out]
            n112 = local write "SCAN QR STATION 2"(w556) -> ()
            n113 = call "debuglog.vi"("Enum"=w552, "Log data"=w553) -> ()  [unwired: 10 in]
          }
          frame "barcode CHECK" {
            # "SCAN OK\tM542\t\t\t2590\nSCAN NG \tM543\t\t\t2591\nSoftware on Bit\tM544\t\t\t2592\nRQST FROM TCO RESET SCAN DATA\tM545\t\t\t2593\nRepeat scan part\t\tM547\t\t2595\nPass not done station 1\t\tM548\t\t2596"
            # "Remove customer\npart n0 from scan QR code"
            # "check QR code from station 1"
            # "VERIFY BARCODE GENERATED IN STATION 1"
            n114 = local read "SCAN QR STATION 2"() -> (w582:string)
            n115 = Unbundle By Name(w584) -> ("connection reference"=w590:T2, "PART_NO"=w583:string)
            n116 = Reverse String(1:w582) -> (0:w581:string)
            n117 = String Subset(string=w581, length (rest)=10 ("length (rest)")) -> (substring=w580:string)  [unwired: 1 in]
            n118 = Reverse String(1:w580) -> (0:w579:string)
            n119 = Equal?(x=w583, y=w579) -> (x = y?=w586:bool)
            n120 = case shown="True" w586 {
              tunnel: w591 -> [w606 w619]
              tunnel: w590 -> [_ w632]
              tunnel: w582 -> [_ w622]
              tunnel: ["Wrong Model QR code on Station 2" ("Cycle Status") w628] -> w589
              tunnel: [Ass._Loop_Control."Wait" ("Enum") w625] -> w588
              tunnel: [w605 w629] -> w585
              tunnel: w584 -> [w597 w624]
              tunnel: [w597 w623] -> w576
              tunnel: w578 -> [w593 w620]
              tunnel: [w593 w616] -> w577
              tunnel: [FALSE w614] -> w574
              frame False {
                # "SCAN OK\tM542\t\t\t2590\nSCAN NG \tM543\t\t\t2591\nSoftware on Bit\tM544\t\t\t2592\nRQST FROM TCO RESET SCAN DATA\tM545\t\t\t2593\nRepeat scan part\t\tM547\t\t2595\nPass not done station 1\t\tM548\t\t2596"
                # "SCAN OK\nSCAN NG \nSoftware on Bit\nRQST FRM TCO REST SCN DT"
                n121 = call "TAT_LABVIEW_TO_PLC_St2.vi"("Enum"=enum16{"Read", "Write"}."Read", "error in (no error)"=w606) -> ("error out"=w600:errorcluster, "Array 2"=w599:bool[])  [unwired: 8 in]
                n122 = in-place {
                  in-place-border: [w613] -> w601
                  in-place-border: w600 -> [w613]
                  w611 = FALSE ("new element/subarray")
                  n123 = in-place-array #2(w599, 0, 1, 3, 4, 5) -> ()  [unwired: 5 out]
                  n124 = in-place-array #2(w611, TRUE ("element"), w611, w611, w611) -> (w598:bool[])  [unwired: 5 out]
                }
                n125 = local write "SCAN QR STATION 2"("" ("SCAN QR STATION 2")) -> ()
                n126 = call "TAT_LABVIEW_TO_PLC_St2.vi"("Enum"=enum16{"Read", "Write"}."Write", "error in (no error)"=w601, "Array"=w598) -> ("error out"=w605:errorcluster)  [unwired: 7 in, 1 out]
              }
              frame True {
                n127 = call <vilib>:"Acquire Semaphore.vi"("error in (no error)"=w619, "semaphore"=w620) -> ("error out"=w618:errorcluster, "semaphore out"=w617:T9)  [unwired: 3 in, 1 out]
                n128 = call "QR_code_Check_St2.vi"("Columns"=string[] ["Station1_QR", "Station2_Rst"] ("columns 2"), "error in (no error)"=w618, "replace %s"=w622, "table"="dbo.Data_Log", "Refnum in"=w632) -> ("error out"=w615:errorcluster, "FALSE healty"=w627:bool, "TRUE Duplication on Station 2"=w626:bool)  [unwired: 1 in, 3 out]
                n129 = call <vilib>:"Clear Errors.vi"("error in (no error)"=w615) -> ("error out"=w621:errorcluster)  [unwired: 5 in, 1 out]
                n130 = call <vilib>:"Release Semaphore.vi"("error in (no error)"=w621, "semaphore"=w617) -> ("semaphore out"=w616:T9)  [unwired: 4 in, 1 out]
                n131 = case shown="False" w627 {
                  tunnel: ["QR OK" ("Cycle Status") w675] -> w628
                  tunnel: w615 -> [w643 w668]
                  tunnel: [w642 w667] -> w629
                  tunnel: w626 -> [_ w663]
                  tunnel: [Ass._Loop_Control."Wait" ("Enum") Ass._Loop_Control."Wait" ("Enum")] -> w625
                  tunnel: w624 -> [w638 w661]
                  tunnel: [w637 w661] -> w623
                  tunnel: w622 -> [w636 _]
                  tunnel: [TRUE FALSE] -> w614
                  frame False {
                    # "Set PLC bit to OK QR & cycle ready to Start"
                    n132 = call "TAT_LABVIEW_TO_PLC_St2.vi"("Enum"=enum16{"Read", "Write"}."Read", "error in (no error)"=w643) -> ("error out"=w650:errorcluster, "Array 2"=w644:bool[])  [unwired: 8 in]
                    n133 = in-place {
                      in-place-border: [w654] -> w649
                      in-place-border: w650 -> [w654]
                      w652 = FALSE ("element")
                      n134 = in-place-array #3(w644, 0, 1, 3, 4, 5) -> ()  [unwired: 5 out]
                      n135 = in-place-array #3(TRUE ("new element/subarray"), w652, w652, w652, w652) -> (w647:bool[])  [unwired: 5 out]
                    }
                    n136 = Bundle By Name(cluster=w638, "Station1_QR"=w636) -> (w637:T5)
                    n137 = call "TAT_LABVIEW_TO_PLC_St2.vi"("Enum"=enum16{"Read", "Write"}."Write", "error in (no error)"=w649, "Array"=w647) -> ("error out"=w642:errorcluster)  [unwired: 7 in, 1 out]
                  }
                  frame True {
                    n138 = call "TAT_LABVIEW_TO_PLC_St2.vi"("Enum"=enum16{"Read", "Write"}."Read", "error in (no error)"=w668) -> ("error out"=w674:errorcluster, "Array 2"=w669:bool[])  [unwired: 8 in]
                    n139 = case shown="False" w663 {
                      tunnel: ["No part gone through station 1" "Part repeated on Station 2" ("Cycle Status")] -> w675
                      tunnel: [FALSE ("new element/subarray") TRUE ("new element/subarray")] -> w658
                      tunnel: [TRUE ("new element/subarray") FALSE ("new element/subarray")] -> w657
                      frame False {
                      }
                      frame True {
                      }
                    }
                    n140 = local write "SCAN QR STATION 2"("" ("SCAN QR STATION 2")) -> ()
                    n141 = in-place {
                      in-place-border: [w686] -> w673
                      in-place-border: w674 -> [w686]
                      in-place-border: w658 -> [w683]
                      in-place-border: w657 -> [w682]
                      w684 = FALSE ("element")
                      n142 = in-place-array #4(w669, 0, 1, 3, 4, 5) -> ()  [unwired: 5 out]
                      n143 = in-place-array #4(FALSE ("new element/subarray"), w684, w684, w683, w682) -> (w672:bool[])  [unwired: 5 out]
                    }
                    n144 = call "TAT_LABVIEW_TO_PLC_St2.vi"("Enum"=enum16{"Read", "Write"}."Write", "error in (no error)"=w673, "Array"=w672) -> ("error out"=w667:errorcluster)  [unwired: 7 in, 1 out]
                  }
                }
              }
            }
            n145 = local write "CYCLE STATUS STATION 2"(w589) -> ()
            n146 = Bundle By Name(cluster=w576, "SearchBitInterlck"=w574) -> (w575:T5)
          }
          frame "Start Cycle" {
            w687 = enum16{"update", "init"}."update"  # Enum
            w688 = "cycle start"  # Log data
            # "SCAN OK\tM542\t\t\t2590\nSCAN NG \tM543\t\t\t2591\nSoftware on Bit\tM544\t\t\t2592\nRQST FROM TCO RESET SCAN DATA\tM545\t\t\t2593\nRepeat scan part\t\tM547\t\t2595\nPass not done station 1\t\tM548\t\t2596"
            n147 = control-ref of="CYCLE STATUS STATION 2"() -> (w705:refnum<vi>)
            n148 = call "STATION_2_STATUS.vi"("error in (no error)"=w704, "STATUS"="CYCLE STARTED" ("Cycle Status"), "Ctl Refnum"=w705) -> ("error out"=w690:errorcluster)  [unwired: 8 in]
            n149 = call "debuglog.vi"("Enum"=w687, "Log data"=w688) -> ()  [unwired: 10 in]
            n150 = call "TAT_LABVIEW_TO_PLC_St2.vi"("Enum"=enum16{"Read", "Write"}."Read", "error in (no error)"=w690) -> ("error out"=w701:errorcluster, "Array 2"=w696:bool[])  [unwired: 8 in]
            n151 = in-place {
              in-place-border: [w709] -> w700
              in-place-border: w701 -> [w709]
              w708 = FALSE ("new element/subarray")
              n152 = in-place-array #5(w696, 0, 1, 3, 4, 5) -> ()  [unwired: 5 out]
              n153 = in-place-array #5(w708, w708, w708, w708, w708) -> (w698:bool[])  [unwired: 5 out]
            }
            n154 = call "TAT_LABVIEW_TO_PLC_St2.vi"("Enum"=enum16{"Read", "Write"}."Write", "error in (no error)"=w700, "Array"=w698) -> ("error out"=w689:errorcluster)  [unwired: 7 in, 1 out]
          }
          frame "GENERATE_QR_PRNT" {
            w710 = enum16{"update", "init"}."update"  # Enum
            w711 = "report saved"  # Log data
            w713 = u32 0  # milliseconds to wait
            # "SCAN BYPASS---2598\nRQS TO TCO READ SCAN DATA \n\nCYCLE START (RUNNING CYCLE)\nCYCLE STOP\nCYCLE COMPLETE\n--45325\nby pass station 1 Bit\nStation 1 valid BIT"
            # "GENERATE QR CODE AND PRINT QR CODE"
            n155 = call "Stall Data Flow.vim"("value in"=w715, "milliseconds to wait"=w713) -> ("value out"=w714:errorcluster)  [unwired: 1 out]
            n156 = call "TAT_PLC_Data_read_BOLLEAN_St2.vi"("Enum"=enum16{"Read", "Write"}."Read", "error in (no error)"=w714) -> ("error out"=w721:errorcluster, "Array 2"=w723:bool[])  [unwired: 8 in]
            n157 = Index Array(array=w723, index=6) -> (element=w720:bool)
            n158 = call "NEW_PRN Generation_Station2.vi"("error in (no error)"=w721, "ClusterIN"=w725) -> ("error out"=w716:errorcluster, "ClusterOUT"=w718:T11, "QR CODE"=w726:string)  [unwired: 7 in]
            n159 = case shown="False" w720 {
              tunnel: w726 -> [_ w732]
              tunnel: [w728 w732] -> w719
              tunnel: [w729 w731] -> w717
              tunnel: w718 -> [w730 w731]
              frame False {
                # "QR not need as done on station 1"
                n160 = local read "SCAN QR STATION 2"() -> (w728:string)
                n161 = Bundle By Name(cluster=w730, "Station2_QR"=w728) -> (w729:T11)
              }
              frame True {
                # "Station 1 bypass"
              }
            }
            n162 = local write "QR STATION 2"(w719) -> ()
            n163 = call "debuglog.vi"("Enum"=w710, "Log data"=w711) -> ()  [unwired: 10 in]
          }
          frame "SaveReport " {
            # "Save Barcode code AND RESULT in SQL"
            n164 = call "TAT_PLC_Data_read_BOLLEAN_St2.vi"("Enum"=enum16{"Read", "Write"}."Read", "error in (no error)"=w744) -> ("error out"=w737:errorcluster, "Array 2"=w742:bool[])  [unwired: 8 in]
            n165 = Index Array(array=w742, index=6) -> (element=w740:bool)
            n166 = call <vilib>:"Acquire Semaphore.vi"("error in (no error)"=w737, "semaphore"=w735) -> ("error out"=w736:errorcluster, "semaphore out"=w734:T9)  [unwired: 3 in, 1 out]
            n167 = case shown="True" w740 {
              tunnel: w736 -> [w750 w753]
              tunnel: [w749 w752] -> w738
              tunnel: w745 -> [w748 w751]
              frame False {
                # "All Station done"
                n168 = Unbundle By Name(w748) -> ("Station1_QR"=w747:string)
                n169 = call "Station2_Data_Log.vi"("error in (no error)"=w750, "Station_QR"=w747, "Cluster 2"=w748) -> ("error out"=w749:errorcluster)  [unwired: 8 in]
              }
              frame True {
                # "Station 1 bypass"
                n170 = call "Station2_Data_Log_Bypass_Station1.vi"("error in (no error)"=w753, "Cluster 2"=w751) -> ("error out"=w752:errorcluster)  [unwired: 9 in]
              }
            }
            n171 = call <vilib>:"Clear Errors.vi"("error in (no error)"=w738) -> ("error out"=w739:errorcluster)  [unwired: 5 in, 1 out]
            n172 = call <vilib>:"Release Semaphore.vi"("error in (no error)"=w739, "semaphore"=w734) -> ("semaphore out"=w733:T9)  [unwired: 4 in, 1 out]
          }
          frame "Cycle End" {
            # "SCAN OK\tM542\t\t\t2590\nSCAN NG \tM543\t\t\t2591\nSoftware on Bit\tM544\t\t\t2592\nRQST FROM TCO RESET SCAN DATA\tM545\t\t\t2593\nRepeat scan part\t\tM547\t\t2595\nPass not done station 1\t\tM548\t\t2596"
            n173 = call "TAT_LABVIEW_TO_PLC_St2.vi"("Enum"=enum16{"Read", "Write"}."Read", "error in (no error)"=w765) -> ("error out"=w774:errorcluster, "Array 2"=w769:bool[])  [unwired: 8 in]
            n174 = in-place {
              in-place-border: [w780] -> w773
              in-place-border: w774 -> [w780]
              w779 = FALSE ("new element/subarray")
              n175 = in-place-array #6(w769, 0, 1, 3, 4, 5) -> ()  [unwired: 5 out]
              n176 = in-place-array #6(w779, w779, TRUE ("new element/subarray"), w779, w779) -> (w771:bool[])  [unwired: 5 out]
            }
            n177 = local write "SCAN QR STATION 2"("" ("SCAN QR STATION 2")) -> ()
            n178 = call "TAT_LABVIEW_TO_PLC_St2.vi"("Enum"=enum16{"Read", "Write"}."Write", "error in (no error)"=w773, "Array"=w771) -> ("error out"=w758:errorcluster)  [unwired: 7 in, 1 out]
            n179 = Bundle By Name(cluster=w755, "SearchBitInterlck"=FALSE) -> (w754:T5)
            n180 = flat-sequence {
              tunnel: [w777] -> w761
              tunnel: w758 -> [w777]
              frame #0 {
                n181 = global write "Global 1.vi" "Station 2 Cycle cmplt"(TRUE) -> ()
              }
            }
            n182 = control-ref of="CYCLE STATUS STATION 2"() -> (w760:refnum<vi>)
            n183 = call "STATION_2_STATUS.vi"("error in (no error)"=w758, "STATUS"="CYCLE END" ("Cycle Status"), "Ctl Refnum"=w760) -> ()  [unwired: 8 in, 1 out]
          }
          frame "Stop" {
            w781 = enum16{"update", "init"}."update"  # Enum
            w782 = "application stop"  # Log data
            # "Clean All bits."
            n184 = control-ref of="CYCLE STATUS STATION 2"() -> (w801:refnum<vi>)
            n185 = call "STATION_2_STATUS.vi"("error in (no error)"=w799, "STATUS"="STOP" ("TexT"), "Ctl Refnum"=w801) -> ("error out"=w798:errorcluster)  [unwired: 8 in]
            n186 = call <vilib>:"Clear Errors.vi"("error in (no error)"=w798) -> ("error out"=w784:errorcluster)  [unwired: 5 in, 1 out]
            n187 = call "TAT_LABVIEW_TO_PLC_St2.vi"("Enum"=enum16{"Read", "Write"}."Read", "error in (no error)"=w784) -> ("error out"=w796:errorcluster, "Array 2"=w789:bool[])  [unwired: 8 in]
            n188 = in-place {
              in-place-border: [w806] -> w797
              in-place-border: w796 -> [w806]
              w804 = FALSE ("element")
              n189 = in-place-array #7(w789, 0, 1, 2, 3, 4, 5) -> ()  [unwired: 6 out]
              n190 = in-place-array #7(FALSE ("new element/subarray"), w804, w804, w804, w804, w804) -> (w794:bool[])  [unwired: 6 out]
            }
            n191 = call "TAT_LABVIEW_TO_PLC_St2.vi"("Enum"=enum16{"Read", "Write"}."Write", "error in (no error)"=w797, "Array"=w794) -> ("error out"=w785:errorcluster)  [unwired: 7 in, 1 out]
            n192 = call "debuglog.vi"("Enum"=w781, "Log data"=w782) -> ()  [unwired: 10 in]
          }
        }
      }
      frame Error {
        w811 = T7 1 items=["no dialog", "OK message", "continue or stop message", "OK message + warnings", "continue/stop + warnings"] ("type of dialog (OK msg:1)")
        w813 = Ass._Loop_Control."Stop"  # Enum
        n193 = call <vilib>:"Simple Error Handler.vi"("type of dialog (OK msg:1)"=w811, "error in (no error)"=w810) -> ("error out"=w809:errorcluster)  [unwired: 3 in, 4 out]
        n194 = call <vilib>:"Clear Errors.vi"("error in (no error)"=w809) -> ("error out"=w808:errorcluster)  [unwired: 5 in, 1 out]
      }
    }
    n195 = case shown="No Error" w157 {
      selector: w157 -> [w199 w455]
      tunnel: w185 -> [w204 _]
      tunnel: w184 -> [w203 w452]
      tunnel: [w202 w452] -> w183
      tunnel: [w201 w453] -> w171
      tunnel: [w200 w451] -> w163
      tunnel: w146 -> [w198 w454]
      tunnel: [w197 w454] -> w145
      tunnel: [_ TRUE] -> w140
      frame No Error {
        n196 = case "Station 3" shown="\"Waiting_for_scan\", Default" w204 {
          tunnel: [Ass._Loop_Control."Cluster_update" ("Enum") Ass._Loop_Control."Waiting_for_scan" ("Enum") w263 w306 w358 Ass._Loop_Control."SaveReport " ("Enum") Ass._Loop_Control."Cycle End" ("Enum") Ass._Loop_Control."Waiting_for_scan" ("Enum") Ass._Loop_Control."Stop" ("Enum") Ass._Loop_Control."Wait" ("Enum")] -> w201
          tunnel: [w218 w226 w262 w312 w357 w403 w420 w438 w442 w446] -> w202
          tunnel: [w212 w232 w256 w310 w364 w395 w407 w422 w441 w447] -> w200
          tunnel: w199 -> [w208 w248 w258 w311 w370 w391 w415 w435 w441 w447]
          tunnel: w203 -> [w217 w242 w262 w313 w357 w400 w417 w438 w442 w446]
          tunnel: w198 -> [w205 w220 w257 w300 w353 w381 w411 w436 w440 w445]
          tunnel: [w205 w220 w257 w299 w353 w381 w410 w436 w440 w445] -> w197
          frame "Int" {
            # "1. INT\n2.CLUSTER UPDATE\n3. WAIT FOR SCAN\n4. BARCODE CHECK AND VERIFY\n\n4.GENERATE AND PRINT QR CODE\n5.SAVE REPORT\n6.CYCLE END\n7.GO TO STEP 3"
            # "Initialize STATION 2"
            n197 = call "TAT_PLC_Data_read.vi"("Enum"=enum16{"Read", "Write"}."Read", "error in (no error)"=w208) -> ("error out"=w207:errorcluster, "Array 2"=w210:u16[])  [unwired: 8 in]
            n198 = Index Array(array=w210) -> ()  [unwired: 1 in, 1 out]
            n199 = Unbundle By Name(w217) -> ("Varient path"=w206:path)
            n200 = call <vilib>:"Open Config Data.vi"("error in (no error)"=w207, "configuration file path"=w206) -> ("error out"=w215:errorcluster, "refnum"=w216:T12)  [unwired: 7 in, 1 out]
            n201 = call <vilib>:"Get Section Names.vi"("error in (no error)"=w215, "refnum"=w216) -> ("error out"=w214:errorcluster, "section names"=w211:string[], "refnum out"=w213:T12)  [unwired: 7 in]
            n202 = call <vilib>:"Close Config Data.vi"("error in (no error)"=w214, "refnum"=w213) -> ("error out"=w212:errorcluster)  [unwired: 8 in, 1 out]
            n203 = Bundle By Name(cluster=w217, "Part Name List"=w211) -> (w218:T3)
          }
          frame "Cluster_update" {
            w224 = "" ("Barcode station 2 to log")
            w225 = string[] [] ("PREVIOUS Code")
            # "Update cluster if varient change"
            n204 = Unbundle By Name(w242) -> ("Varient path"=w223:path, "Part Name List"=w239:string[])
            n205 = local read "Model Selection:-"() -> (w237:string)
            n206 = Search 1D Array(1D array=w239, element=w237) -> (index of element=w241:i32)  [unwired: 1 in]
            n207 = Increment(x=w241) -> (x+1=w238:i32)
            n208 = call "Varient_number_check.vi"("Varient No."=w238, "Varient path"=w223, "error in"=w248) -> ("TORISHI_CODE"=w247:string, "Part Name"=w246:string, "Varient Number"=w235:i32, "STATION 1 BYPASS"=w221:bool, "Batch Size"=w230:i32, "MODEL LIST"=w240:string[], "PART_NO"=w245:string, "error out"=w243:errorcluster)  [unwired: 4 in, 1 out]
            "Station 1 Bypass" <- w221
            n209 = Number To Decimal String(number=w230) -> (decimal integer string=→"PACKAGE Qty":string)  [unwired: 1 in]
            n210 = First Call?() -> (First Call?: T/F=w236:bool)
            n211 = Bundle By Name(cluster=w242, "Station 1 bypass"=w221, "TORISHI_CODE"=w247, "Part name"=w246, "Varient number"=w235, "Batch_Size"=w230, "PART_NO"=w245, "Part Name List"=w240) -> (w227:T3)
            n212 = case shown="True" w236 {
              tunnel: w243 -> [w250 w253]
              tunnel: [w250 w252] -> w233
              tunnel: w240 -> [_ w251]
              frame False {
              }
              frame True {
                n213 = property on="Model Selection:-" class="CmbBox"(error in=w253, "Strings[]"=w251) -> (error out=w252:errorcluster)  [unwired: 1 in, 1 out]
              }
            }
            n214 = Unbundle By Name(w227) -> ("Current Varient path"=w231:path)
            n215 = call "Varient_Current_Status.vi"("Enum"=enum16{"Write", "Read"}."Write", "error in"=w233, "Current Varient Status"=w231, "Batch Size"=w230, "Varient count"=0) -> ("error out"=w232:errorcluster)  [unwired: 4 in, 2 out]
            n216 = Bundle By Name(cluster=w227, "PREVIOUS code"=w225, "Station 2 barcode Dn"=w224, "Station 2 barcode Up"=w224) -> (w226:T3)
            n217 = local write "PREVIOUS BARCODE 2"(w225) -> ()
            n218 = local write "Scanned Qty  2"("") -> ()
            n219 = local write "BARCODE STATION 3"("") -> ()
          }
          frame "Waiting_for_scan", Default {
            w254 = 10.0  # Time Target (s)
            # "WATING FOR SCAN"
            n220 = local read "Model Selection:-"() -> (w260:string)
            n221 = Unbundle By Name(w262) -> ("Part name"=w261:string)
            n222 = Equal?(x=w261, y=w260) -> (x = y?=w259:bool)
            n223 = case shown="True" w259 {
              tunnel: [w269 w281] -> w256
              tunnel: [Ass._Loop_Control."Cluster_update" ("Enum") w280] -> w263
              tunnel: w258 -> [w269 w271]
              tunnel: w262 -> [_ _]
              frame False {
              }
              frame True {
                n224 = local read "BARCODE STATION 3"() -> (w279:string)
                n225 = String Length(string=w279) -> (length=w278:i32)
                n226 = Greater?(x=w278, y=2) -> (0:w276:bool)
                n227 = case shown="True" w276 {
                  tunnel: w271 -> [w288 w291]
                  tunnel: [w288 w290] -> w273
                  frame False {
                  }
                  frame True {
                    n228 = call "Stall Data Flow.vim"("value in"=w291, "milliseconds to wait"=u32 2000) -> ("value out"=w290:errorcluster)  [unwired: 1 out]
                  }
                }
                n229 = flat-sequence {
                  tunnel: [w284] -> w275
                  tunnel: [w283] -> w274
                  tunnel: w273 -> [w283]
                  tunnel: [w282] -> w272
                  frame #0 {
                    n230 = local read "BARCODE STATION 3"() -> (w282:string)
                    n231 = String Length(string=w282) -> (length=w287:i32)
                    n232 = In Range and Coerce(upper limit=50 ("y"), x=w287, lower limit=30) -> (In Range?=w284:bool)  [unwired: 1 out]
                  }
                }
                n233 = case shown="True" w275 {
                  tunnel: w274 -> [w294 w298]
                  tunnel: [w294 w298] -> w281
                  tunnel: [Ass._Loop_Control."Waiting_for_scan" ("Enum") Ass._Loop_Control."barcode CHECK" ("Enum")] -> w280
                  tunnel: w272 -> [_ w296]
                  frame False {
                    # "SCAN DONE - SET PLC BIT\n TO READY CYCLE"
                    # "SET PLC BIT TO INDICATE SCAN DONE"
                    n234 = local write "BARCODE STATION 3"("") -> ()
                  }
                  frame True {
                    n235 = call <vilib>:"Trim Whitespace.vi"("string"=w296) -> ("trimmed string"=w295:string)  [unwired: 1 in]
                    n236 = local write "BARCODE STATION 3"(w295) -> ()
                  }
                }
              }
            }
            n237 = call "Elapsed Time"("Time Target (s)"=w254) -> ("Time has Elapsed"=w255:bool)  [unwired: 11 in, 7 out]
            n238 = case shown="True" w255 {
              tunnel: w256 -> [_ w264]
              frame False {
              }
              frame True {
                n239 = control-ref of="This VI"() -> (w265:refnum<vi>)
                n240 = property class="VI"(reference=w265, error in=w264, "Front Panel.IsFrontmost"=TRUE) -> (error out=w268:errorcluster)  [unwired: 1 out]
                n241 = property on="BARCODE STATION 3" class="Str"(error in=w268, "Key Focus"=TRUE) -> ()  [unwired: 1 in, 2 out]
              }
            }
          }
          frame "barcode CHECK" {
            # "verify local duplication\n&\ncorrect Part No"
            # "check QR code from station 1"
            # "VERIFY BARCODE GENERATED IN STATION 1 and station 2"
            n242 = Unbundle By Name(w313) -> ("Station 1 bypass"=w301:bool, "PREVIOUS code"=w305:string[], "connection reference"=w309:T2, "PART_NO"=w308:string)
            n243 = local read "BARCODE STATION 3"() -> (w304:string)
            n244 = call "Station3_QR_Code_correct&localduplication_verification.vi"("BARCODE STATION in"=w304, "PART_NO"=w308, "PRIVIOUS code"=w305) -> ("Correct part no True"=w302:bool, "Correct part no & No duplication TRUE"=w303:bool)  [unwired: 7 in]
            n245 = case shown="True" w303 {
              tunnel: w313 -> [w319 w339]
              tunnel: [w319 w338] -> w312
              tunnel: w311 -> [w318 w328]
              tunnel: [w318 w325] -> w310
              tunnel: w309 -> [_ w337]
              tunnel: w304 -> [_ w332]
              tunnel: [w317 w334] -> w307
              tunnel: [Ass._Loop_Control."Cycle End" ("Enum") w333] -> w306
              tunnel: w302 -> [w315 _]
              tunnel: w301 -> [_ w329]
              tunnel: w300 -> [w314 w326]
              tunnel: [w314 w322] -> w299
              frame False {
                n246 = case shown="True" w315 {
                  tunnel: ["Wrong Model QR code on Station 3" ("Cycle Status") "Duplicate QR code on Station 3" ("Cycle Status")] -> w317
                  frame False {
                  }
                  frame True {
                  }
                }
              }
              frame True {
                n247 = call <vilib>:"Acquire Semaphore.vi"("error in (no error)"=w328, "semaphore"=w326) -> ("error out"=w327:errorcluster, "semaphore out"=w323:T9)  [unwired: 3 in, 1 out]
                n248 = call "QR_code_Check_St3.vi"("Columns"=string[] ["Station2_QR", "Station3_Rst"] ("columns 2"), "Station 1 Bypass"=w329, "error in (no error)"=w327, "replace %s"=w332, "table"="dbo.Data_Log", "Refnum in"=w337) -> ("error out"=w325:errorcluster, "FALSE healty"=w331:bool, "TRUE Duplication on Station 2"=w330:bool)  [unwired: 2 out]
                n249 = case shown="True" w331 {
                  tunnel: ["QR OK" ("Cycle Status") w350] -> w334
                  tunnel: w339 -> [w343 w349]
                  tunnel: [w345 w349] -> w338
                  tunnel: [Ass._Loop_Control."Package_Qty_Count" ("Enum") Ass._Loop_Control."Cycle End" ("Enum")] -> w333
                  tunnel: w332 -> [w340 _]
                  tunnel: w330 -> [_ w347]
                  frame False {
                    n250 = Unbundle By Name(w343) -> ("PREVIOUS code"=w342:string[])
                    n251 = Build Array (concatenate)(w342, w340) -> (w341:string[])
                    n252 = Bundle By Name(cluster=w343, "PREVIOUS code"=w341) -> (w345:T3)
                  }
                  frame True {
                    n253 = case shown="True" w347 {
                      tunnel: ["No part gone through station 2" ("Cycle Status") "Part repeated on Station 3" ("Cycle Status")] -> w350
                      frame False {
                      }
                      frame True {
                      }
                    }
                  }
                }
                n254 = call <vilib>:"Clear Errors.vi"("error in (no error)"=w325) -> ("error out"=w324:errorcluster)  [unwired: 5 in, 1 out]
                n255 = call <vilib>:"Release Semaphore.vi"("error in (no error)"=w324, "semaphore"=w323) -> ("semaphore out"=w322:T9)  [unwired: 4 in, 1 out]
              }
            }
            n256 = local write "CYCLE STATUS STATION 3"(w307) -> ()
          }
          frame "Package_Qty_Count" {
            # "Count packaged scanned qr code"
            n257 = Unbundle By Name(w357) -> ("Current Varient path"=w356:path)
            n258 = call "Varient_Current_Status.vi"("Enum"=enum16{"Write", "Read"}."Read", "error in"=w370, "Current Varient Status"=w356) -> ("error out"=w368:errorcluster, "Batch Size"=w361:i32, "Varient Count"=w367:i32)  [unwired: 6 in]
            n259 = Increment(x=w367) -> (x+1=w362:i32)
            n260 = Equal?(x=w362, y=w361) -> (x = y?=w366:bool)
            n261 = case shown="False" w366 {
              tunnel: [w375 w380] -> w363
              tunnel: w368 -> [w375 w380]
              tunnel: w362 -> [w372 _]
              tunnel: w361 -> [w374 w379]
              tunnel: [w374 w379] -> w360
              tunnel: [w372 0] -> w359
              tunnel: [Ass._Loop_Control."Cycle End" ("Enum") Ass._Loop_Control."GENERATE_QR_PRNT" ("Enum")] -> w358
              tunnel: [w371 "" ("String")] -> w355
              frame False {
                # "incnt part count."
                n262 = Number To Decimal String(number=w372) -> (decimal integer string=w371:string)  [unwired: 1 in]
              }
              frame True {
                # "Batch pack qty cmplt--- Print Package slip"
              }
            }
            "Scanned Qty  2" <- w355
            n263 = Unbundle By Name(w357) -> ("PREVIOUS code"=→"PREVIOUS BARCODE 2":string[])
            n264 = call "Varient_Current_Status.vi"("Enum"=enum16{"Write", "Read"}."Write", "error in"=w363, "Current Varient Status"=w356, "Batch Size"=w360, "Varient count"=w359) -> ("error out"=w364:errorcluster)  [unwired: 4 in, 2 out]
          }
          frame "GENERATE_QR_PRNT" {
            # "printer COMMUNICATION"
            # "Save PACKAGE Barcode code AND RESULT in SQL"
            n265 = Unbundle By Name(w400) -> ("Package path"=w404:path)
            n266 = local write "CYCLE STATUS STATION 3"("PACKAGING BARCODE PRINTED" ("Cycle Status")) -> ()
            n267 = call "PRN Generation_Station_2.vi"("error in (no error)"=w391, "PRN path"=w404, "Cluster"=w400) -> ("error out"=w392:errorcluster, "Barcode Station 2 Up"=w401:string, "Barcode station 2 Dn"=w402:string, "PRN to Print"=w385:string)  [unwired: 2 in]
            "PRN to Print" <- w385
            n268 = Bundle By Name(cluster=w400, "Station 2 barcode Up"=w401, "Station 2 barcode Dn"=w402) -> (w403:T3)
            n269 = Open/Create/Replace File(file path (use dialog)=path "C:/Users/Admin/NIVision/STATION2.prn", error in=w392, operation (0:open)=T10."replace or create") -> (refnum out=w386:refnum<file>, error out=w387:errorcluster)  [unwired: 3 in, 1 out]
            n270 = Write to Text File(file (use dialog)=w386, text=w385, error in=w387) -> (refnum out=w388:refnum<file>, error out=w389:errorcluster)  [unwired: 1 in, 1 out]
            n271 = Close File(refnum=w388, error in=w389) -> (error out=w384:errorcluster)  [unwired: 1 out]
            n272 = call "Stall Data Flow.vim"("value in"=w384, "milliseconds to wait"=u32 2000) -> ("value out"=w383:errorcluster)  [unwired: 1 out]
            n273 = call <vilib>:"System Exec.vi"("run minimized? (F)"=FALSE, "error in (no error)"=w383, "working directory"=path "C:/", "standard input"="COPY / B C:\\Users\\Admin\\NIVision\\STATION2.prn \\\\Tataficosa\\ZDesign\n", "command line"="cmd") -> ("error out"=w396:errorcluster)  [unwired: 3 in, 3 out]
            n274 = Merge Errors(w392, w396) -> (w395:errorcluster)
          }
          frame "SaveReport " {
            w418 = "" ("Barcode station 2 to log")
            w419 = string[] [] ("PREVIOUS Code")
            # "Save Barcode code AND RESULT in SQL"
            n275 = call <vilib>:"Acquire Semaphore.vi"("error in (no error)"=w415, "semaphore"=w411) -> ("error out"=w414:errorcluster, "semaphore out"=w412:T9)  [unwired: 3 in, 1 out]
            n276 = call "Station3_Data_Log.vi"("Cluster"=w417, "error in (no error)"=w414) -> ("error out"=w408:errorcluster)  [unwired: 8 in]
            n277 = call <vilib>:"Clear Errors.vi"("error in (no error)"=w408) -> ("error out"=w413:errorcluster)  [unwired: 5 in, 1 out]
            n278 = call <vilib>:"Release Semaphore.vi"("error in (no error)"=w413, "semaphore"=w412) -> ("semaphore out"=w410:T9)  [unwired: 4 in, 1 out]
            n279 = call "Stall Data Flow.vim"("value in"=w408, "milliseconds to wait"=u32 2000) -> ("value out"=w407:errorcluster)  [unwired: 1 out]
            n280 = Bundle By Name(cluster=w417, "PREVIOUS code"=w419, "Station 2 barcode Dn"=w418, "PREVIOUS code"=w419, "Station 2 barcode Up"=w418) -> (w420:T3)
            n281 = local write "PREVIOUS BARCODE 2"(w419) -> ()
            n282 = local write "BARCODE STATION 3"("") -> ()
          }
          frame "Cycle End" {
            w434 = u32 0 ("dy")
            # "Sets cursor position"
            # "Gets cursor position"
            # "Clicks left mouse button"
            # "Sets cursor position"
            n283 = local write "BARCODE STATION 3"("") -> ()
            n284 = call <vilib>:"Clear Errors.vi"("error in (no error)"=w435) -> ("error out"=w422:errorcluster)  [unwired: 5 in, 1 out]
            n285 = dll-call lib="User32.dll" fn="GetCursorPos" ("Move mouse to new pos")(error in=w422) -> (error out=w427:errorcluster, "POINT"=w430:i32[])  [unwired: 4 in, 1 out]
            n286 = control-ref of="BARCODE STATION 3"() -> (w423:refnum<vi>)
            n287 = property on="Property Node" class="Str"(reference=w423, error in=w427) -> (error out=w426:errorcluster, "Left"=w429:i32, "Top"=w428:i32)  [unwired: 1 out]
            n288 = dll-call lib="User32.dll" fn="SetCursorPos" ("Move mouse to new pos")(error in=w426, "dx"=w429, "dy"=w428) -> (error out=w431:errorcluster)  [unwired: 5 in, 1 out]
            n289 = dll-call lib="user32.dll" fn="mouse_event"(error in=w431, "dwFlags"=u32 2, "dx"=w434, "dy"=w434, "dwData"=w434, "dwExtraInfo"=w434) -> (error out=w433:errorcluster)  [unwired: 8 in, 1 out]
            n290 = Index Array(array=w430) -> (element #1=w424:i32, element #2=w425:i32)  [unwired: 2 in]
            n291 = dll-call lib="User32.dll" fn="SetCursorPos" ("Move mouse to new pos")(error in=w433, "dx"=w424, "dy"=w425) -> ()  [unwired: 5 in, 2 out]
          }
          frame "Stop" {
            n292 = local write "CYCLE STATUS STATION 3"("STATION STOP" ("Cycle Status")) -> ()
          }
          frame "Start Cycle" {
            n293 = local write "CYCLE STATUS STATION 1"("Cycle started" ("Cycle Status")) -> ()
          }
        }
      }
      frame Error {
        w453 = Ass._Loop_Control."Stop"  # Enum
        w457 = T7 1 items=["no dialog", "OK message", "continue or stop message", "OK message + warnings", "continue/stop + warnings"] ("type of dialog (OK msg:1)")
        n294 = call <vilib>:"Simple Error Handler.vi"("type of dialog (OK msg:1)"=w457, "error in (no error)"=w455) -> ("error out"=w456:errorcluster)  [unwired: 3 in, 4 out]
        n295 = call <vilib>:"Clear Errors.vi"("error in (no error)"=w456) -> ("error out"=w451:errorcluster)  [unwired: 5 in, 1 out]
      }
    }
    n296 = case shown="No Error" w139 {
      selector: w139 -> [w818 w1170]
      tunnel: w196 -> [w823 _]
      tunnel: w194 -> [w822 w1167]
      tunnel: [w821 _] -> w186
      tunnel: [w820 Ass._Loop_Control."Stop" ("Enum")] -> w181
      tunnel: [w819 w1167] -> w180
      tunnel: [w817 w1165] -> w152
      tunnel: w150 -> [w816 w1168]
      tunnel: [w815 w1168] -> w149
      tunnel: [_ TRUE] -> w143
      frame No Error {
        n297 = case "Station 1" shown="\"Wait\", Default" w823 {
          tunnel: [Ass._Loop_Control."Cluster_update" ("Enum") Ass._Loop_Control."Wait" ("Enum") w887 Ass._Loop_Control."Wait" ("Enum") w950 Ass._Loop_Control."Wait" ("Enum") Ass._Loop_Control."Wait" ("Enum") Ass._Loop_Control."SaveReport " ("Enum") Ass._Loop_Control."Cycle End" ("Enum") Ass._Loop_Control."Wait" ("Enum") Ass._Loop_Control."Stop" ("Enum")] -> w820
          tunnel: [w840 w851 w885 w939 w945 w1001 w1070 w1081 w1099 w1117 w1157] -> w819
          tunnel: w822 -> [w840 w852 w885 w939 w946 w1002 w1070 w1087 w1099 w1118 w1157]
          tunnel: [_ _ _ _ _ _ _ _ _ _ TRUE] -> w821
          tunnel: [w831 w857 w873 w903 w948 w1014 w1057 w1086 w1092 w1119 w1155] -> w817
          tunnel: w818 -> [w843 w861 w883 w924 w974 w1018 w1069 w1089 w1107 w1132 w1158]
          tunnel: w816 -> [w830 w848 w870 w938 w962 w1011 w1068 w1080 w1096 w1121 w1141]
          tunnel: [w830 w848 w870 w938 w962 w1010 w1068 w1080 w1094 w1121 w1141] -> w815
          frame "Int" {
            w828 = "initia"  # Log data
            w829 = enum16{"update", "init"}."init"  # Enum
            # "SCAN OK\nSCAN NG \nSoftware on Bit\nRQST FROM TCO RESET SCAN DATA\nRepeat scan part\t\tM547"
            # "1. INT\n2.CLUSTER UPDATE\n3. WAIT\n4.GENERATE AND PRINT QR CODE\n5.SAVE REPORT\n6.CYCLE END\n7.GO TO STEP 3"
            # "Initialize"
            n298 = control-ref of="CYCLE STATUS STATION 1"() -> (w842:refnum<vi>)
            n299 = call "STATION_1_STATUS.vi"("error in (no error)"=w843, "STATUS"="STATION 7A - EOL - 1" ("TexT"), "Ctl Refnum"=w842) -> ("error out"=w832:errorcluster)  [unwired: 8 in]
            n300 = call "TAT_LABVIEW_TO_PLC.vi"("Enum"=enum16{"Read", "Write"}."Read", "error in (no error)"=w832) -> ("error out"=w838:errorcluster, "Array 2"=w833:bool[])  [unwired: 8 in]
            n301 = in-place {
              in-place-border: [w847] -> w839
              in-place-border: w838 -> [w847]
              w845 = FALSE ("new element/subarray")
              w846 = TRUE ("new element/subarray")
              # "Software on,\nrqst to reset Bit"
              n302 = in-place-array #8(w833, 0, 1, 2, 3, 4) -> ()  [unwired: 5 out]
              n303 = in-place-array #8(w845, w845, w846, w846, w845) -> (w836:bool[])  [unwired: 5 out]
            }
            n304 = call "TAT_LABVIEW_TO_PLC.vi"("Enum"=enum16{"Read", "Write"}."Write", "error in (no error)"=w839, "Array"=w836) -> ("error out"=w831:errorcluster)  [unwired: 7 in, 1 out]
            n305 = call "debuglog2.vi"("Enum"=w829, "Log data"=w828) -> ()  [unwired: 10 in]
          }
          frame "Cluster_update" {
            # "CYCLE TIME\nAMBIENT TEMP\nBLINKER CURRENT OK\nTEMP SENSOR OK\nPART OK COUNT\nPART NOK COUNT\nFAULT BIT\nVARIENT\nHOUR\nMINUTE\nSECOND\nDAY\nMONTH\nYEAR\nSERIAL NUMBER"
            # "PART NAME\nPART No.\nPACKAGE QUANTITY\nTORISHI CODE"
            # "PART NAME---\nVARIENT NAME"
            # "Update cluster if varient change"
            n306 = call "TAT_PLC_Data_read.vi"("Enum"=enum16{"Read", "Write"}."Read", "error in (no error)"=w861) -> ("error out"=w858:errorcluster, "Array 2"=w863:u16[])  [unwired: 8 in]
            n307 = Index Array(array=w863, index=7) -> (element=w854:u16)
            n308 = Unbundle By Name(w852) -> ("Varient path"=w855:path)
            n309 = call "Varient_number_check.vi"("Varient No."=w854, "Varient path"=w855, "error in"=w858) -> ("HARNESS_CODE"=w849:string, "TORISHI_CODE"=w853:string, "Part Name"=w860:string, "Batch Size"=w856:i32, "PART_NO"=w859:string, "error out"=w857:errorcluster)  [unwired: 4 in, 3 out]
            "PART No.:-" <- w859
            "TORISHI CODE:-" <- w853
            "HARNESS CODE" <- w849
            n310 = local write "PART NAME :-"(w860) -> ()
            n311 = Bundle By Name(cluster=w852, "Part name"=w860, "Varient number"=w854, "Batch_Size"=w856, "PART_NO"=w859, "TORISHI_CODE"=w853, "Harness_QR_code"=w849) -> (w851:T6)
          }
          frame "Wait", Default {
            w884 = enum16{"Read", "Write"}."Read" ("Enum")
            # "CYCLE TIME\nAMBIENT TEMP\nBLINKER CURRENT OK\nTEMP SENSOR OK\nPART OK COUNT\nPART NOK COUNT\nFAULT BIT\nVARIENT\nHOUR\nMINUTE\nSECOND\nDAY\nMONTH\nYEAR\nSERIAL NUMBER"
            # "BLINKER CURRENT OK\nTEMP SENSOR OK\nAVM OK\nIV3 CAMERA OK SIGNAL\nCYCLE COMPLETE\nCYCLE START (RUNNING CYCLE)\nCYCLE STOP\nSCAN BYPASS\nRQS TO TCO READ SCAN DATA"
            # "WAITING FORM CCYLE TO COMPLE TO PRINT QR"
            # "Wait"
            n312 = Unbundle By Name(w885) -> ("SearchBitInterlck"=w866:bool, "Varient number"=w888:u16)
            n313 = call "TAT_PLC_Data_read.vi"("Enum"=w884, "error in (no error)"=w883) -> ("error out"=w874:errorcluster, "Array 2"=w889:u16[])  [unwired: 8 in]
            n314 = call "TAT_PLC_Data_read_BOLLEAN.vi"("Enum"=w884, "error in (no error)"=w883) -> ("error out"=w872:errorcluster, "Array 2"=w882:bool[])  [unwired: 8 in]
            n315 = Index Array(array=w889, index=7) -> (element=w890:u16)
            n316 = Index Array(array=w882, index #1=4 ("index")) -> (element #1=w879:bool, element #2=w880:bool, element #3=w878:bool, element #4=w867:bool, element #5=w871:bool)  [unwired: 4 in]
            n317 = Merge Errors(w874, w872) -> (w873:errorcluster)
            n318 = Not Equal?(x=w888, y=w890) -> (x != y?=w886:bool)
            n319 = Or(x=w866, y=w867) -> (x .or. y?=w865:bool)
            n320 = call <userlib>:"Boolean Trigger__ogtk.vi"("Boolean Input"=w879) -> ("Rising Edge"=w868:bool)  [unwired: 1 in, 1 out]
            n321 = call <userlib>:"Boolean Trigger__ogtk.vi"("Boolean Input"=w878) -> ("Rising Edge"=w877:bool)  [unwired: 1 in, 1 out]
            n322 = call <userlib>:"Boolean Trigger__ogtk.vi"("Boolean Input"=w880) -> ("Rising Edge"=w893:bool)  [unwired: 1 in, 1 out]
            n323 = call <userlib>:"Boolean Trigger__ogtk.vi"("Boolean Input"=w871) -> ("Rising Edge"=w876:bool)  [unwired: 1 in, 1 out]
            n324 = And(x=w865, y=w868) -> (x .and. y?=w869:bool)
            n325 = Build Array(w893, w869, w886, w877, w876) -> (w892:bool[])
            n326 = Search 1D Array(1D array=w892, element=TRUE ("Boolean Input")) -> (index of element=w891:i32)  [unwired: 1 in]
            n327 = case shown="1" w891 {
              tunnel: [Ass._Loop_Control."frontpanel Display update" ("Enum") Ass._Loop_Control."Start Cycle" ("Enum") Ass._Loop_Control."GENERATE_QR_PRNT" ("Enum") Ass._Loop_Control."Cluster_update" ("Enum") Ass._Loop_Control."Cycle End" ("Enum") Ass._Loop_Control."Waiting_for_scan" ("Enum")] -> w887
              frame -1, Default {
              }
              frame 0 {
                # "CYCYLE START BIT"
              }
              frame 1 {
                # "CYCLE cmpt STORE RLT"
              }
              frame 2 {
                # "CLUSTER UPDATE"
              }
              frame 3 {
                w899 = "direct cycle stop"  # Log data
                w900 = enum16{"update", "init"}."update"  # Enum
                # "Cycle Stop/Cancle."
                # "cycle stop / E stop"
                n328 = call "debuglog2.vi"("Enum"=w900, "Log data"=w899) -> ()  [unwired: 10 in]
              }
              frame 4 {
                # "wait for scaning"
              }
            }
          }
          frame "frontpanel Display update" {
            # "\"frontpanel Display update\""
            n329 = control-ref of="CYCLE STATUS STATION 1"() -> (w928:refnum<vi>)
            n330 = call "TAT_PLC_Data_read.vi"("Enum"=enum16{"Read", "Write"}."Read", "error in (no error)"=w924) -> ("error out"=w923:errorcluster, "Array 2"=w931:u16[])  [unwired: 8 in]
            n331 = Index Array(array=w931, index #2=6 ("index")) -> (element #1=→"CYCLE TIME:-":u16, element #2=w930:u16)  [unwired: 1 in]
            n332 = call "STATION_1_STATUS.vi"("error in (no error)"=w923, "FAULT NUMBER"=w930, "Ctl Refnum"=w928) -> ("error out"=w904:errorcluster)  [unwired: 8 in]
            n333 = Index Array(array=w931, index #1=19 ("index")) -> (element #1=w932:u16, element #2=w933:u16, element #5=w934:u16, element #6=w935:u16, element #7=w936:u16)  [unwired: 6 in, 2 out]
            n334 = local write "BLINKER CURRENT MIN"(w932) -> ()
            n335 = local write "BLINKER CURRENT MAX"(w933) -> ()
            n336 = local write "TEMP SENSOR MIN"(w934) -> ()
            n337 = local write "TEMP SENSOR MAX"(w935) -> ()
            n338 = local write "AMBIET TEMP MIN"(w936) -> ()
            n339 = call "TAT_PLC_Data_read_BOLLEAN.vi"("Enum"=enum16{"Read", "Write"}."Read", "error in (no error)"=w904) -> ("error out"=w903:errorcluster, "Array 2"=w908:bool[])  [unwired: 8 in]
            n340 = Index Array(array=w908, index #5=4 ("index"), index #7=9 ("index")) -> (element #1=w911:bool, element #2=w912:bool, element #3=w913:bool, element #4=w914:bool, element #5=→"CYCLE RESULT:-":bool, element #6=→"CYCLE START:-":bool, element #7=w915:bool, element #8=w916:bool, element #9=w917:bool, element #10=w918:bool, element #11=w919:bool, element #12=w920:bool, element #13=w921:bool, element #14=w922:bool)  [unwired: 12 in]
            n341 = local write "Blinker ct st1"(w911) -> ()
            n342 = local write "Temp Sensor st1"(w912) -> ()
            n343 = local write "PY1B LHD RH PART SENSOR"(w918) -> ()
            n344 = local write "PY1B RHD RH PART SENSOR"(w919) -> ()
            n345 = local write "HBC RH PART SENSOR"(w920) -> ()
            n346 = local write "PY1B LHD LH PART SENSOR"(w915) -> ()
            n347 = local write "PY1B RHD LH PART SENSOR"(w916) -> ()
            n348 = local write "HBC LH PART SENSOR"(w917) -> ()
            n349 = local write "AVM St1"(w913) -> ()
            n350 = local write "iv3 camera st1"(w914) -> ()
            n351 = local write "RAREJECTION BIN"(w921) -> ()
            n352 = local write "PRINT LABEL PICKUP"(w922) -> ()
          }
          frame "Waiting_for_scan" {
            w941 = "search bit rcv"  # Log data
            w947 = enum16{"update", "init"}."update"  # Enum
            w956 = "\t"
            # "remove harness number from scan data"
            # "Compare scaned harness QR with recipe Harness code"
            # "Harness QR code to read"
            # "Scanne Data from PLC register"
            n353 = call "Station 1 QR Code.vi"("Enum"=enum16{"Read", "Write"}."Read", "error in (no error)"=w974) -> ("error out"=w949:errorcluster, "Array 2"=w975:u16[])  [unwired: 8 in]
            n354 = Type Cast(type="", x=w975) -> (*(type *) &x=w964:string)
            n355 = String Subset(string=w964, length (rest)=49 ("length (rest)")) -> (substring=w963:string)  [unwired: 1 in]
            n356 = Unbundle By Name(w946) -> ("Harness_QR_code"=w952:string)
            n357 = call <vilib>:"Space Constant.vi"() -> ("String"=w967:string)
            n358 = Search and Replace String(replace all?=TRUE ("replace all? (F)"), input string=w963, search string="[^a-zA-Z0-9]", replace string=w967) -> (result string=w966:string)  [unwired: 4 in, 3 out]
            n359 = call <vilib>:"Trim Whitespace.vi"("string"=w966) -> ("trimmed string"=w965:string)  [unwired: 1 in]
            n360 = Search and Replace String(replace all?=TRUE ("replace all? (F)"), input string=w965, search string="  ", replace string=" " ("search string")) -> (result string=w942:string)  [unwired: 4 in, 3 out]
            n361 = call <vilib>:"Space Constant.vi"() -> ("String"=w961:string)
            n362 = local write "QR STATION 1"(w942) -> ()
            n363 = Search and Replace String(replace all?=TRUE ("replace all? (F)"), input string=w942, search string=w961, replace string=w956) -> (result string=w960:string)  [unwired: 4 in, 3 out]
            n364 = Concatenate Strings(w941, " ", w942) -> (w940:string)
            n365 = Spreadsheet String To Array(delimiter (Tab)=w956, format string="", spreadsheet string=w960, array type (2D Dbl)=string[] []) -> (array=w959:string[])
            n366 = Index Array(array=w959, index=0) -> (element=w958:string)
            n367 = call "debuglog2.vi"("Enum"=w947, "Log data"=w940) -> ()  [unwired: 10 in]
            n368 = Equal?(x=w952, y=w958) -> (x = y?=w951:bool)
            n369 = case shown="False" w951 {
              tunnel: [w991 Ass._Loop_Control."barcode CHECK" ("Enum")] -> w950
              tunnel: w949 -> [w980 w998]
              tunnel: [w979 w998] -> w948
              tunnel: [FALSE TRUE] -> w944
              frame False {
                w991 = Ass._Loop_Control."Wait"  # Enum
                # "SCAN OK\nSCAN NG \nSoftware on Bit\nRQST FROM TCO RESET SCAN DATA\nRepeat scan part\t\tM547"
                n370 = call "TAT_LABVIEW_TO_PLC.vi"("Enum"=enum16{"Read", "Write"}."Read", "error in (no error)"=w980) -> ("error out"=w990:errorcluster, "Array 2"=w981:bool[])  [unwired: 8 in]
                n371 = in-place {
                  in-place-border: [w996] -> w989
                  in-place-border: w990 -> [w996]
                  w994 = FALSE ("new element/subarray")
                  n372 = in-place-array #9(w981, 0, 1, 3, 4) -> ()  [unwired: 4 out]
                  n373 = in-place-array #9(w994, TRUE ("element"), w994, w994) -> (w987:bool[])  [unwired: 4 out]
                }
                n374 = control-ref of="CYCLE STATUS STATION 1"() -> (w993:refnum<vi>)
                n375 = call "STATION_1_STATUS.vi"("STATUS"="Wrong Model QR code on Station 1" ("Cycle Status"), "Ctl Refnum"=w993) -> ()  [unwired: 9 in, 1 out]
                n376 = call "TAT_LABVIEW_TO_PLC.vi"("Enum"=enum16{"Read", "Write"}."Write", "error in (no error)"=w989, "Array"=w987) -> ("error out"=w979:errorcluster)  [unwired: 7 in, 1 out]
              }
              frame True {
              }
            }
            n377 = Bundle By Name(cluster=w946, "SearchBitInterlck"=w944) -> (w945:T6)
          }
          frame "barcode CHECK" {
            # "SCAN OK\nSCAN NG \nSoftware on Bit\nRQST FROM TCO RESET SCAN DATA\nRepeat scan part\t\tM547"
            # "Harness scan code"
            # "check QR code from station 1"
            n378 = Unbundle By Name(w1002) -> ("connection reference"=w1019:T2)
            n379 = local read "QR STATION 1"() -> (w1012:string)
            n380 = call <vilib>:"Acquire Semaphore.vi"("error in (no error)"=w1018, "semaphore"=w1011) -> ("error out"=w1006:errorcluster, "semaphore out"=w1005:T9)  [unwired: 3 in, 1 out]
            n381 = call "QR_code_Check_St1.vi"("Columns"=string[] ["Harness_QR_St1"] ("columns 2"), "error in (no error)"=w1006, "replace %s"=w1012, "table"="dbo.Data_Log", "Refnum in"=w1019) -> ("error out"=w1003:errorcluster, "TRUE no barcode Done on station 1"=w1007:bool)  [unwired: 1 in, 3 out]
            n382 = call <vilib>:"Clear Errors.vi"("error in (no error)"=w1003) -> ("error out"=w1004:errorcluster)  [unwired: 5 in, 1 out]
            n383 = call <vilib>:"Release Semaphore.vi"("error in (no error)"=w1004, "semaphore"=w1005) -> ("semaphore out"=w1010:T9)  [unwired: 4 in, 1 out]
            n384 = case shown="True" w1007 {
              tunnel: ["Part repeated on Station 1" ("Cycle Status") "QR OK" ("Cycle Status")] -> w1015
              tunnel: w1003 -> [w1026 w1042]
              tunnel: [w1025 w1041] -> w1013
              tunnel: [FALSE TRUE] -> w1000
              frame False {
                n385 = call "TAT_LABVIEW_TO_PLC.vi"("Enum"=enum16{"Read", "Write"}."Read", "error in (no error)"=w1026) -> ("error out"=w1032:errorcluster, "Array 2"=w1027:bool[])  [unwired: 8 in]
                n386 = in-place {
                  in-place-border: [w1036] -> w1031
                  in-place-border: w1032 -> [w1036]
                  w1034 = FALSE ("new element/subarray")
                  n387 = in-place-array #10(w1027, 0, 1, 3, 4) -> ()  [unwired: 4 out]
                  n388 = in-place-array #10(w1034, w1034, w1034, TRUE ("element")) -> (w1030:bool[])  [unwired: 4 out]
                }
                n389 = call "TAT_LABVIEW_TO_PLC.vi"("Enum"=enum16{"Read", "Write"}."Write", "error in (no error)"=w1031, "Array"=w1030) -> ("error out"=w1025:errorcluster)  [unwired: 7 in, 1 out]
              }
              frame True {
                # "Set PLC bit to OK QR & cycle ready to Start"
                n390 = call "TAT_LABVIEW_TO_PLC.vi"("Enum"=enum16{"Read", "Write"}."Read", "error in (no error)"=w1042) -> ("error out"=w1049:errorcluster, "Array 2"=w1043:bool[])  [unwired: 8 in]
                n391 = in-place {
                  in-place-border: [w1053] -> w1048
                  in-place-border: w1049 -> [w1053]
                  w1051 = FALSE ("element")
                  n392 = in-place-array #11(w1043, 0, 1, 3, 4) -> ()  [unwired: 4 out]
                  n393 = in-place-array #11(TRUE ("new element/subarray"), w1051, w1051, w1051) -> (w1046:bool[])  [unwired: 4 out]
                }
                n394 = call "TAT_LABVIEW_TO_PLC.vi"("Enum"=enum16{"Read", "Write"}."Write", "error in (no error)"=w1048, "Array"=w1046) -> ("error out"=w1041:errorcluster)  [unwired: 7 in, 1 out]
              }
            }
            n395 = control-ref of="CYCLE STATUS STATION 1"() -> (w1016:refnum<vi>)
            n396 = Bundle By Name(cluster=w1002, "SearchBitInterlck"=w1000) -> (w1001:T6)
            n397 = call "STATION_1_STATUS.vi"("error in (no error)"=w1013, "STATUS"=w1015, "Ctl Refnum"=w1016) -> ("error out"=w1014:errorcluster)  [unwired: 8 in]
          }
          frame "Start Cycle" {
            w1066 = "cycle start"  # Log data
            w1067 = enum16{"update", "init"}."update"  # Enum
            # "SCAN OK\nSCAN NG \nSoftware on Bit\nRQST FROM TCO RESET SCAN DATA\nRepeat scan part\t\tM547"
            n398 = control-ref of="CYCLE STATUS STATION 1"() -> (w1072:refnum<vi>)
            n399 = call "STATION_1_STATUS.vi"("error in (no error)"=w1069, "STATUS"="CYCLE STARTED" ("Cycle Status"), "Ctl Refnum"=w1072) -> ("error out"=w1058:errorcluster)  [unwired: 8 in]
            n400 = call "debuglog2.vi"("Enum"=w1067, "Log data"=w1066) -> ()  [unwired: 10 in]
            n401 = call "TAT_LABVIEW_TO_PLC.vi"("Enum"=enum16{"Read", "Write"}."Read", "error in (no error)"=w1058) -> ("error out"=w1064:errorcluster, "Array 2"=w1060:bool[])  [unwired: 8 in]
            n402 = in-place {
              in-place-border: [w1075] -> w1065
              in-place-border: w1064 -> [w1075]
              w1074 = FALSE ("new element/subarray")
              # "Software on,\nrqst to reset Bit"
              n403 = in-place-array #12(w1060, 0, 1, 3, 4) -> ()  [unwired: 4 out]
              n404 = in-place-array #12(w1074, w1074, w1074, w1074) -> (w1063:bool[])  [unwired: 4 out]
            }
            n405 = call "TAT_LABVIEW_TO_PLC.vi"("Enum"=enum16{"Read", "Write"}."Write", "error in (no error)"=w1065, "Array"=w1063) -> ("error out"=w1057:errorcluster)  [unwired: 7 in, 1 out]
          }
          frame "GENERATE_QR_PRNT" {
            w1078 = "report saved"  # Log data
            w1079 = enum16{"update", "init"}."update"  # Enum
            # "CYCLE TIME\nAMBIENT TEMP\nBLINKER CURRENT OK\nTEMP SENSOR OK\nPART OK COUNT\nPART NOK COUNT\nFAULT BIT\nVARIENT\nHOUR\nMINUTE\nSECOND\nDAY\nMONTH\nYEAR\nSERIAL NUMBER\nShift\nAVM\nTS\nIV3"
            # "GENERATE QR CODE AND QR CODE"
            n406 = call "TAT_PLC_Data_read.vi"("Enum"=enum16{"Read", "Write"}."Read", "error in (no error)"=w1089) -> ("error out"=w1088:errorcluster, "Array 2"=w1090:u16[])  [unwired: 8 in]
            n407 = Index Array(array=w1090) -> (element #2=w1084:u16, element #3=w1083:u16, element #4=w1082:u16)  [unwired: 4 in, 1 out]
            n408 = call "NEW_PRN Generation_Station1.vi"("error in (no error)"=w1088, "ClusterIN"=w1087) -> ("error out"=w1086:errorcluster, "ClusterOUT"=w1081:T13)  [unwired: 8 in]
            n409 = local write "AMBIENT TEMP st 1"(w1084) -> ()
            n410 = local write "BLINKER CURRENT OK st 1"(w1083) -> ()
            n411 = local write "TEMP SENSOR st 1"(w1082) -> ()
            n412 = Unbundle By Name(w1081) -> ("Station1_QR"=w1076:string)
            n413 = local write "QR STATION 3"(w1076) -> ()
            n414 = Concatenate Strings(w1078, " ", w1076) -> ()  [unwired: 1 out]
            n415 = call "debuglog2.vi"("Enum"=w1079, "Log data"=w1078) -> ()  [unwired: 10 in]
          }
          frame "SaveReport " {
            # "Save Barcode code AND RESULT in SQL"
            n416 = Unbundle By Name(w1099) -> ("Current Serial Number"=w1114:string)
            n417 = local read "BLINKER CURRENT OK st 1"() -> (w1110:u32)
            n418 = call "TAT_PLC_Data_read_BOLLEAN.vi"("Enum"=enum16{"Read", "Write"}."Read" ("Enum 2"), "error in (no error)"=w1107) -> ("error out"=w1098:errorcluster, "Array 2"=w1105:bool[])  [unwired: 8 in]
            n419 = local read "AMBIENT TEMP st 1"() -> (w1111:u32)
            n420 = local read "TEMP SENSOR st 1"() -> (w1109:u32)
            n421 = local read "QR STATION 1"() -> (w1102:string)
            n422 = Index Array(array=w1105, index=7) -> (element=w1103:bool)
            n423 = Decimal String To Number(string=w1114, default (0L)=u32 0 ("default (0 I32)")) -> (number=→"SERIAL NO.:- 2":u32)  [unwired: 1 in, 1 out]
            n424 = Select(t="Harness_QR_Bypass", s=w1103, f=w1102) -> (s? t:f=w1101:string)
            n425 = call <vilib>:"Acquire Semaphore.vi"("error in (no error)"=w1098, "semaphore"=w1096) -> ("error out"=w1097:errorcluster, "semaphore out"=w1095:T9)  [unwired: 3 in, 1 out]
            n426 = Bundle("QR STATION 1"=w1101, "AMBIENT TEMP st 1"=w1111, "BLINKER CURRENT OK st 1"=w1110, "TEMP SENSOR st 1"=w1109) -> (w1108:T14)  [unwired: 1 in]
            n427 = call "Station1_Data_Log.vi"("error in (no error)"=w1097, "Parameters cluster"=w1108, "Cluster"=w1099) -> ("error out"=w1092:errorcluster)  [unwired: 8 in]
            n428 = call <vilib>:"Clear Errors.vi"("error in (no error)"=w1092) -> ("error out"=w1093:errorcluster)  [unwired: 5 in, 1 out]
            n429 = call <vilib>:"Release Semaphore.vi"("error in (no error)"=w1093, "semaphore"=w1095) -> ("semaphore out"=w1094:T9)  [unwired: 4 in, 1 out]
          }
          frame "Cycle End" {
            w1116 = FALSE  # searchbitinterlck
            # "SCAN OK\nSCAN NG \nSoftware on Bit\nRQST FROM TCO RESET SCAN DATA\nRepeat scan part\t\tM547"
            n430 = call "TAT_LABVIEW_TO_PLC.vi"("Enum"=enum16{"Read", "Write"}."Read", "error in (no error)"=w1132) -> ("error out"=w1131:errorcluster, "Array 2"=w1124:bool[])  [unwired: 8 in]
            n431 = in-place {
              in-place-border: [w1138] -> w1130
              in-place-border: w1131 -> [w1138]
              w1137 = FALSE ("new element/subarray")
              n432 = in-place-array #13(w1124, 0, 1, 3, 4) -> ()  [unwired: 4 out]
              n433 = in-place-array #13(w1137, w1137, TRUE ("new element/subarray"), w1137) -> (w1128:bool[])  [unwired: 4 out]
            }
            n434 = call "TAT_LABVIEW_TO_PLC.vi"("Enum"=enum16{"Read", "Write"}."Write", "error in (no error)"=w1130, "Array"=w1128) -> ("error out"=w1120:errorcluster)  [unwired: 7 in, 1 out]
            n435 = Bundle By Name(cluster=w1118, "SearchBitInterlck"=w1116) -> (w1117:T6)
            n436 = flat-sequence {
              tunnel: [w1135] -> w1119
              tunnel: w1120 -> [w1135]
              frame #0 {
                n437 = global write "Global 1.vi" "Station 1 Cycle cmplt"(TRUE) -> ()
              }
            }
          }
          frame "Stop" {
            w1139 = "application stop"  # Log data
            w1140 = enum16{"update", "init"}."update"  # Enum
            # "SCAN OK.\nSCAN NG .\nSoftware on Bit.\nRQST FRM TCO REST SCN DT.\nPart repeated."
            n438 = control-ref of="CYCLE STATUS STATION 1"() -> (w1160:refnum<vi>)
            n439 = call "STATION_1_STATUS.vi"("error in (no error)"=w1158, "STATUS"="STOP" ("Cycle Status"), "Ctl Refnum"=w1160) -> ("error out"=w1156:errorcluster)  [unwired: 8 in]
            n440 = call <vilib>:"Clear Errors.vi"("error in (no error)"=w1156) -> ("error out"=w1143:errorcluster)  [unwired: 5 in, 1 out]
            n441 = call "TAT_LABVIEW_TO_PLC.vi"("Enum"=enum16{"Read", "Write"}."Read", "error in (no error)"=w1143) -> ("error out"=w1154:errorcluster, "Array 2"=w1147:bool[])  [unwired: 8 in]
            n442 = in-place {
              in-place-border: [w1164] -> w1153
              in-place-border: w1154 -> [w1164]
              w1163 = FALSE ("new element/subarray")
              n443 = in-place-array #14(w1147, 0, 1, 2, 3, 4) -> ()  [unwired: 5 out]
              n444 = in-place-array #14(w1163, w1163, w1163, w1163, w1163) -> (w1151:bool[])  [unwired: 5 out]
            }
            n445 = call "TAT_LABVIEW_TO_PLC.vi"("Enum"=enum16{"Read", "Write"}."Write", "error in (no error)"=w1153, "Array"=w1151) -> ("error out"=w1142:errorcluster)  [unwired: 7 in, 1 out]
            n446 = Merge Errors(w1142, w1156) -> (w1155:errorcluster)
            n447 = call "debuglog2.vi"("Enum"=w1140, "Log data"=w1139) -> ()  [unwired: 10 in]
          }
        }
      }
      frame Error {
        w1171 = T7 1 items=["no dialog", "OK message", "continue or stop message", "OK message + warnings", "continue/stop + warnings"] ("type of dialog (OK msg:1)")
        n448 = call <vilib>:"Simple Error Handler.vi"("type of dialog (OK msg:1)"=w1171, "error in (no error)"=w1170) -> ("error out"=w1169:errorcluster)  [unwired: 3 in, 4 out]
        n449 = call <vilib>:"Clear Errors.vi"("error in (no error)"=w1169) -> ("error out"=w1165:errorcluster)  [unwired: 5 in, 1 out]
      }
    }
    n450 = call "TAT_PLC_Data_read_Parameters_St2.vi"("Enum"=enum16{"Read", "Write"}."Read", "error in (no error)"=w157) -> ("error out"=w153:errorcluster, "Array 2"=w160:u16[])  [unwired: 8 in]
    n451 = call "TAT_PLC_Data_read_St2.vi"("error in (no error)"=w157) -> ("error out"=w156:errorcluster, "Array 2"=w167:u16[])  [unwired: 9 in]
    n452 = control-ref of="CYCLE STATUS STATION 2"() -> (w168:refnum<vi>)
    n453 = call "Live_Update_Value_indicator.vi"("Value Indicators Ref"=w159, "Array in"=w160, "error out"=w153) -> ()  [unwired: 8 in]
    n454 = Index Array(array=w167, index #1=6 ("index"), index #2=15 ("index")) -> (element #1=w166:u16, element #2=→"SHIFT":u16)
    n455 = call "TAT_PLC_Data_read_BOLLEAN_St2.vi"("Enum"=enum16{"Read", "Write"}."Read", "error in (no error)"=w157) -> ("error out"=w154:errorcluster, "Array 2"=w164:bool[])  [unwired: 8 in]
    n456 = call "STATION_2_STATUS.vi"("error in (no error)"=w156, "FAULT NUMBER"=w166, "Ctl Refnum"=w168) -> ()  [unwired: 8 in, 1 out]
    n457 = call "Live_Update_Bollean_indicator.vi"("error in (no error)"=w154, "Array 2"=w164, "Array"=w158) -> ()  [unwired: 9 in]
    n458 = Merge Errors(w154, w153, w156) -> (w155:errorcluster)
    n459 = flat-sequence {
      tunnel: w155 -> [w1177]
      frame #0 {
        # "STATION 2"
        n460 = call "TAT_PLC_Data_read_St2.vi"("Enum"=enum16{"Read", "Write"}."Read", "error in (no error)"=w1177) -> ("Array 2"=w1176:u16[])  [unwired: 8 in, 1 out]
        n461 = Index Array(array=w1176, index #2=14 ("index")) -> (element #1=→"CYCLE TIME:-St2":u16, element #2=→"SERIAL NO.:- St2":u16)  [unwired: 1 in]
      }
    }
    n462 = local read "BARCODE STATION 3"() -> (→"BARCODE STATION 3 only display":string)
    n463 = global read "Global 1.vi" "PLC Communication STATION 1"() -> (→"PLC STATUS:-":bool)
    n464 = global read "Global 1.vi" "PLC Communication STATION 2"() -> (→"PLC STATUS:- 2":bool)
    n465 = Get Date/Time String(want seconds? (F)=TRUE) -> (date string=w190:string, time string=w189:string)  [unwired: 2 in]
    n466 = Concatenate Strings(w190, "\n", w189) -> (→"DATE/TIME":string)
    n467 = Wait (ms)(milliseconds to wait=u32 100) -> ()  [unwired: 1 out]
    n468 = Compound Arithmetic op=OR("Stop", w143, w141, w140) -> (w142:bool)
    n469 = Select(t=Ass._Loop_Control."Stop" ("Enum"), s=w142, f=w176) -> (s? t:f=w175:T4)
    n470 = Select(t=Ass._Loop_Control."Stop" ("Enum"), s=w142, f=w181) -> (s? t:f=w193:T4)
    n471 = Select(t=Ass._Loop_Control."Stop" ("Enum"), s=w142, f=w171) -> (s? t:f=w182:T4)
  }
  n472 = Merge Errors(w1, w2, w6) -> (w98:errorcluster)
  n473 = Unbundle By Name(w78) -> ("connection reference"=w79:T2)
  n474 = call <vilib>:"Simple Error Handler.vi"("type of dialog (OK msg:1)"=w95, "error in (no error)"=w98) -> ("error out"=w73:errorcluster)  [unwired: 3 in, 4 out]
  "error out" <- w73
  n475 = call <vilib>:"Clear Errors.vi"("error in (no error)"=w73) -> ("error out"=w8:errorcluster)  [unwired: 5 in, 1 out]
  n476 = call <vilib>:"DB Tools Close Connection.vi"("error in (no error)"=w8, "connection reference"=w79) -> ("error out"=w74:errorcluster)  [unwired: 5 in]
  n477 = call <vilib>:"Release Semaphore Reference.vi"("error in (no error)"=w8, "semaphore"=w7) -> ("error out"=w5:errorcluster)  [unwired: 8 in, 1 out]
  n478 = property class="App"() -> ("App.Kind"=w93:T8)  [unwired: 2 in, 2 out]
  n479 = Merge Errors(w73, w74, w5) -> (w75:errorcluster)
  n480 = case shown="\"invalid app kind\", Default" w93 {
    tunnel: w75 -> [_ w1180]
    frame "invalid app kind", Default {
    }
    frame "Run Time System" {
      n481 = call <vilib>:"Clear Errors.vi"("error in (no error)"=w1180) -> ("error out"=w1179:errorcluster)  [unwired: 5 in, 1 out]
      n482 = invoke class="VI" method="FP.Close"(error in=w1179) -> ()  [unwired: 2 in, 3 out]
    }
  }
  "CYCLE STATUS STATION 1" <- ""
  "QR STATION 3" <- ""
  "RESULT STATION 1" <- FALSE ("want seconds? (F)")
  "AVM St1" <- w72
  "iv3 camera st1" <- w72
  "AMBIENT TEMP st 1" <- w59
  "Temp Sensor st1" <- w72
  "BLINKER CURRENT OK st 1" <- w59
  "TEMP SENSOR st 1" <- w59
  "Blinker ct st1" <- w72
  "String" <- "PARAMETERS" ("String")
  "BLINKER CURRENT MIN" <- w59
  "TEMP SENSOR MIN" <- w59
  "BLINKER CURRENT MAX" <- w59
  "TEMP SENSOR MAX" <- w59
  "AMBIET TEMP MIN" <- w59
  "PY1B LHD LH PART SENSOR" <- w58
  "PY1B RHD LH PART SENSOR" <- w58
  "HBC LH PART SENSOR" <- w58
  "PY1B LHD RH PART SENSOR" <- w58
  "PY1B RHD RH PART SENSOR" <- w58
  "HBC RH PART SENSOR" <- w58
  "RAREJECTION BIN" <- w58
  "PRINT LABEL PICKUP" <- w58
  "PY1B LHD LH PART SENSOR 2" <- w57
  "PY1B & HBC RH PART VERI SENSR" <- w57
  "GASKET PRESENT SENSOR 2" <- w57
  "PY1B LHD RH PART SENSOR 2" <- w57
  "PY1B & HBC LH PART VERI SENSR" <- w57
  "GASKET PRESENT SENSOR 1" <- w57
  "RAREJECTION BIN 2" <- w57
  "PRINT LABEL PICKUP 2" <- w57
  "POWER FOLD CURENT st2 MIN" <- w56
  "GROUND st2 MIN" <- w56
  "EXTERNAL (DEG) st2 MIN" <- w56
  "INTERNAL (DEG) sT2 MIN" <- w56
  "SKY st2 3 MIN" <- w56
  "GLASS ACTR CT 2 mA st2 MIN" <- w56
  "GLASS PULL TEST st2 MIN" <- w56
  "POWER FOLD CURENT st2 MAX" <- w56
  "GROUND st2 MAX" <- w56
  "EXTERNAL (DEG) st2 MAX" <- w56
  "INTERNAL (DEG) st2 MAX" <- w56
  "SKY st2  MAX" <- w56
  "GLASS ACTR CT 2 mA st2 MAX" <- w56
  "GLASS ACTR CT 1 mA st2 MIN" <- w56
  "GLASS ACTR CT 1 mA st2 MAX" <- w56
